vi "Scope_x410_2channel_IQ_PID.vi"() -> ()   [LabVIEW 2025]
uses:
  FPGA/DataMode.ctl
  <vilib>/Analysis/4window.llb/windowTd.ctl
  Host/Scope/controls/power_spectrum_unit.ctl
  Host/Scope5782/Scope/controls/5782_trigger_type.ctl
  Host/Scope/controls/Data_calc_mode.ctl
  Host/Scope/controls/Data_display_mode.ctl
  Host/Scope/controls/Graph_references.ctl
  Host/Scope/controls/graph_controls.ctl
  Host/Scope/controls/Channel_select_2fpga.ctl
  FPGA/PID/PID control enabled type.ctl
  <vilib>/userDefined/High Color/nirio_resource_hc.ctl
  Host/Scope/controls/All FP controls.ctl
  Host/Scope/controls/Output scale.ctl
  Host/Scope/controls/host_transfer_speed.ctl
  FPGA/cavity model/Piezo setting.ctl
  Host/Scope/controls/w12 scale.ctl
  Host/Scope/controls/FFT buffer type.ctl
  Host/Communication/Driver/RemoteConnection/RemoteReferences.ctl
  Host/FpgaRef/FpgaRef5761/ClockSource_5761.ctl
  Host/INI files/Settings file IQ PID/SettingsFileIQpid.lvclass
  C:/PXIe/InProgress/source/Host/INI files/Settings file base/SettingsFile.lvclass
  Host/Communication/Driver/RemoteConnection/RemoteConnection.lvclass
  Host/Scope/Scope5782_six_channel/Scope5782_six_channel.lvclass
  C:/PXIe/InProgress/source/Host/Scope/ScopeBase/ScopeBase.lvclass
  FPGA/fpga_settings.ctl
  Host/INI files/Settings file base/Save event.ctl
  Host/Scope/Scope5782_six_channel/Scope5782_six_channel.lvclass/Scope5782_six_channel.ctl
  Host/Scope/controls/ScopeMode.ctl
  Host/FpgaRef/FpgaRefx410/FpgaRefx410.lvclass
  C:/PXIe/InProgress/source/Host/FpgaRef/FpgaRefBase/FpgaRefBase.lvclass
  Host/FpgaRef/FpgaRef5761/FpgaRef5761.lvclass
  Host/Communication/global_stop.vi
  <vilib>/FPGAPlugInAG/USRP-X410/niLvFpga_Open_USRP-X410.vi
  <vilib>/rvi/interface/common/dynamic/niFpgaDynamicAddResources.vi
  <vilib>/Utility/error.llb/Error Cluster From Error Code.vi
  <vilib>/rvi/errors/niLvFpgaAdjustHostInterfaceError.vi
  Host/Communication/response.ctl
  Host/Communication/driver_status.ctl
  <vilib>/rvi/interface/nirviOpenFPGA/nirviOpenFPGA.xnode
  FPGA Bitfiles/FPGAmain_x410_IQ_PID_ek52GLrW3nU.lvbitx
  <vilib>/rvi/interface/nirviReadWriteControl/nirviReadWriteControl.xnode
  <vilib>/rvi/FXPMathLib/FxpInterpret/XNode/nifxpmath_Interpret.xnode
  C:/PXIe/InProgress/source/Host/FpgaRef/FpgaRefx410/FpgaRefx410.lvclass
  C:/PXIe/InProgress/source/Host/Scope/Scope5782_six_channel/Scope5782_six_channel.lvclass
  C:/PXIe/InProgress/source/Host/FpgaRef/FpgaRef5761/FpgaRef5761.lvclass
  Host/Communication/Driver/TcpServerDriver/TcpServerDriver.lvclass
  Host/Scope/ScopeBase/ScopeBase.lvclass
  Host/INI files/Settings file base/SettingsFile.lvclass
  <vilib>/FPGAPlugInAG/PXIe-7975R/niLvFpga_Open_PXIe-7975R.vi
  Host/FpgaRef/FpgaRefBase/FpgaRefBase.lvclass
  FPGA Bitfiles/FPGAmain_5761_zuew0qNtRjU.lvbitx
  NiFpgaLv.dll
  <vilib>/rvi/interface/Simulation/niFpgaSimulationCallBeginRW.vi
  <vilib>/Analysis/NI_AALPro.lvlib
panel:
  in  "Device Name":refnum<k15>="RIO0"
  in  "quench":bool
  out "Lower graph":dbl[][](graph)
  out "Upper graph":dbl[][](graph)
  out "Upper chart":dbl[][](graph)
  in  "Hold plot lower":bool caption="Hold plot"
  in  "Update once lower":bool
  in  "Hold plot upper":bool caption="Hold plot"
  in  "Update once upper":bool
  in  "FFT buffer size":T1
  in  "Transfer speed":T2
  out "All FP controls":T3
  in  "Show buffers":bool
  out "Adaptive FF graph":dbl[][](graph)
  in  "Tab Control":T4(tab)
  in  "b":fxp<+/-,16,2>
  in  "a":fxp<+/-,16,2>
  in  "Fequency [kHz]":dbl format="%#_8g"
  in  "I Feedback":T5
  in  "Ki*T AM":fxp<+/-,32,6> caption="Ki*T"
  in  "Kd/T AM":fxp<+/-,32,11> caption="Kd/T"
  in  "Kp AM":fxp<+/-,32,6> caption="Kp"
  in  "Feedback delay":u32
  in  "Trigger delay":u32
  in  "Acquire samples":u32
  in  "Kp Q":fxp<+/-,32,6> caption="Kp"
  in  "Kd/T  Q":fxp<+/-,32,11> caption="Kd/T"
  in  "Ki*T Q":fxp<+/-,32,6> caption="Ki*T"
  in  "Q Feedback":T5
  in  "Output gain dB":dbl
  in  "Host scale 5761":T6 caption="Host scale"
  in  "Input scale 5761":T6 caption="Input scale"
  in  "Host scale":T6
  in  "Input scale":T6
  in  "Output scale":T6
  in  "ch2 DC offset":dbl caption="DC offset\nChannel 2"
  in  "ch3 DC offset":dbl caption="DC offset\nChannel 3"
  in  "ch0 DC offset 2":dbl caption="DC offset\nChannel 0"
  in  "ch1 DC offset 2":dbl caption="DC offset\nChannel 1"
  in  "ch0 DC offset":dbl caption="DC offset\nChannel 0"
  in  "ch1 DC offset":dbl caption="DC offset\nChannel 1"
  in  "Setpoint":path
  in  "Feed forward":path
  in  "show setpoint":bool
  in  "show feedforward":bool
  in  "Setpoint enabled":bool
  in  "Piezo":T7
  in  "w0":dbl
  in  "Virtual cavity":bool
  in  "K2":dbl
  in  "Q2":dbl
  in  "w2":dbl
  in  "K3":dbl
  in  "Q3":dbl
  in  "w3":dbl
  in  "S":dbl=0.001 min=0.001 max=1000.0 format="%#_12g"
  in  "K1":dbl
  in  "Q1":dbl
  in  "w1":dbl
  in  "R1":dbl
  in  "w12":dbl format="%#_12g"
  in  "Cavity model":bool
  in  "Max output set":dbl min=0.0 max=16383.0
  out "Amp1":fxp<+,16,14>
  in  "Reset Quench Warning":bool
  in  "Measure Tau at Time":u32
  in  "Tau set":fxp<+/-,32,13>
  in  "Enable":bool
  out "Tau [µs]":fxp<+/-,64,26>
  out "Quench_Warning":bool
  out "Tau_set":fxp<+/-,32,13>
  in  "Input delay 5782":u32
  in  "Input delay 5761":u32
  in  "Count to skip 5782, stage 1":u32
  in  "Count to skip 5761, stage 1":u32
  in  "Count to skip 5782, stage 2":u32
  in  "Count to skip 5782, stage 3":u32
  in  "Count to skip 5761, stage 2":u32
  in  "Count to skip 5761, stage 3":u32
  in  "Vfi Vfq LP filter cut off frequency":dbl caption="MHz" min=0.0 max=10000.0
  in  "Vi Vq LP  filter cutoff fequency":dbl caption="MHz" min=0.0 max=10000.0
  in  "ch3 delay":dbl caption="ns" min=0.0 max=10000.0
  in  "ch1 delay":dbl caption="ns" min=0.0 max=10000.0
  in  "dw LP filter cut off frequency":dbl caption="MHz" min=0.0 max=10000.0
  in  "w12 LP  filter cutoff fequency":dbl caption="MHz" min=0.0 max=10000.0
  in  "dw scale":T8
  in  "w12 scale":T8
  in  "w12 - dt":dbl min=100.0 max=10000000.0
  in  "Calculate w12":bool
  in  "w12 - a":dbl format="%#_12g"
  in  "w12 - b":dbl
  in  "5761 resource":T9="PXI2Slot11"
  in  "Output enabled":bool=TRUE
  in  "Output delay delta":dbl(slide) scale=0.0..6.0
  in  "Output delay":dbl(slide) scale=0.0..6.0
  in  "Output mixer fequency [MHz]":dbl
  in  "Trigger":T10
  in  "Mode":T11
  in  "Mixer freq [MHz]":dbl
  in  "Unwrap phase":bool
  in  "#bins":i32=1 min=1 max=16
  in  "Unit":T12
  in  "Window":T13=1 items=["Rectangle"=0, "Hanning"=1, "Hamming"=2, "Blackman-Harris"=3, "Exact Blackman"=4, "Blackman"=5, "Flat Top"=6, "4 Term B-Harris "=7, "7 Term B-Harris"=8, "Low Sidelobe"=9, "Blackman Nuttall"=11, "Triangle"=30, "Bartlett-Hanning"=31, "Bohman"=32, "Parzen"=33, "Welch"=34, "Kaiser"=60, "Dolph-Chebyshev"=61, "Gaussian"=62]
  in  "Chart length":i32=400000
  in  "Trigmode":enum32{"Triggered", "Continuous"}(radio)
  in  "Reference for phase":T14
  in  "Graph_refs":T15
  out "Lower chart":dbl[][](graph)
  in  "Buffer":T17
  in  "Display":T18
  out "stop 2":bool
  in  "Zoom freq X":bool
  in  "Zoom freq Y":bool
  in  "Zoom time Y":bool
  in  "Zoom time X":bool
  in  "Samples per 5782 record":i32
  in  "Phase offset (deg)":dbl
  in  "Fequency [MHz]":dbl format="%#_8g"
  out "freqdata":cluster{"f0":dbl, "df":dbl, "magnitude":dbl[]}[](graph)
  in  "Rumode":bool
  in  "Singleshot":bool
  out "error IO":errorcluster
  in  "stop":bool
  # "FPGA setup"
  # "ns"
  # "Output delay"
  # "Auto Zoom"
  # "FFT"
  # "Auto Zoom"
  # "Delays"
  # "Amplitude modulation"
  # "x410"
  # "5761"
  # "5782"
  # "V"
  # "V"
  # "5761"
  # "V"
  # "V"
  # "V"
  # "V"
  # "Simulated data"
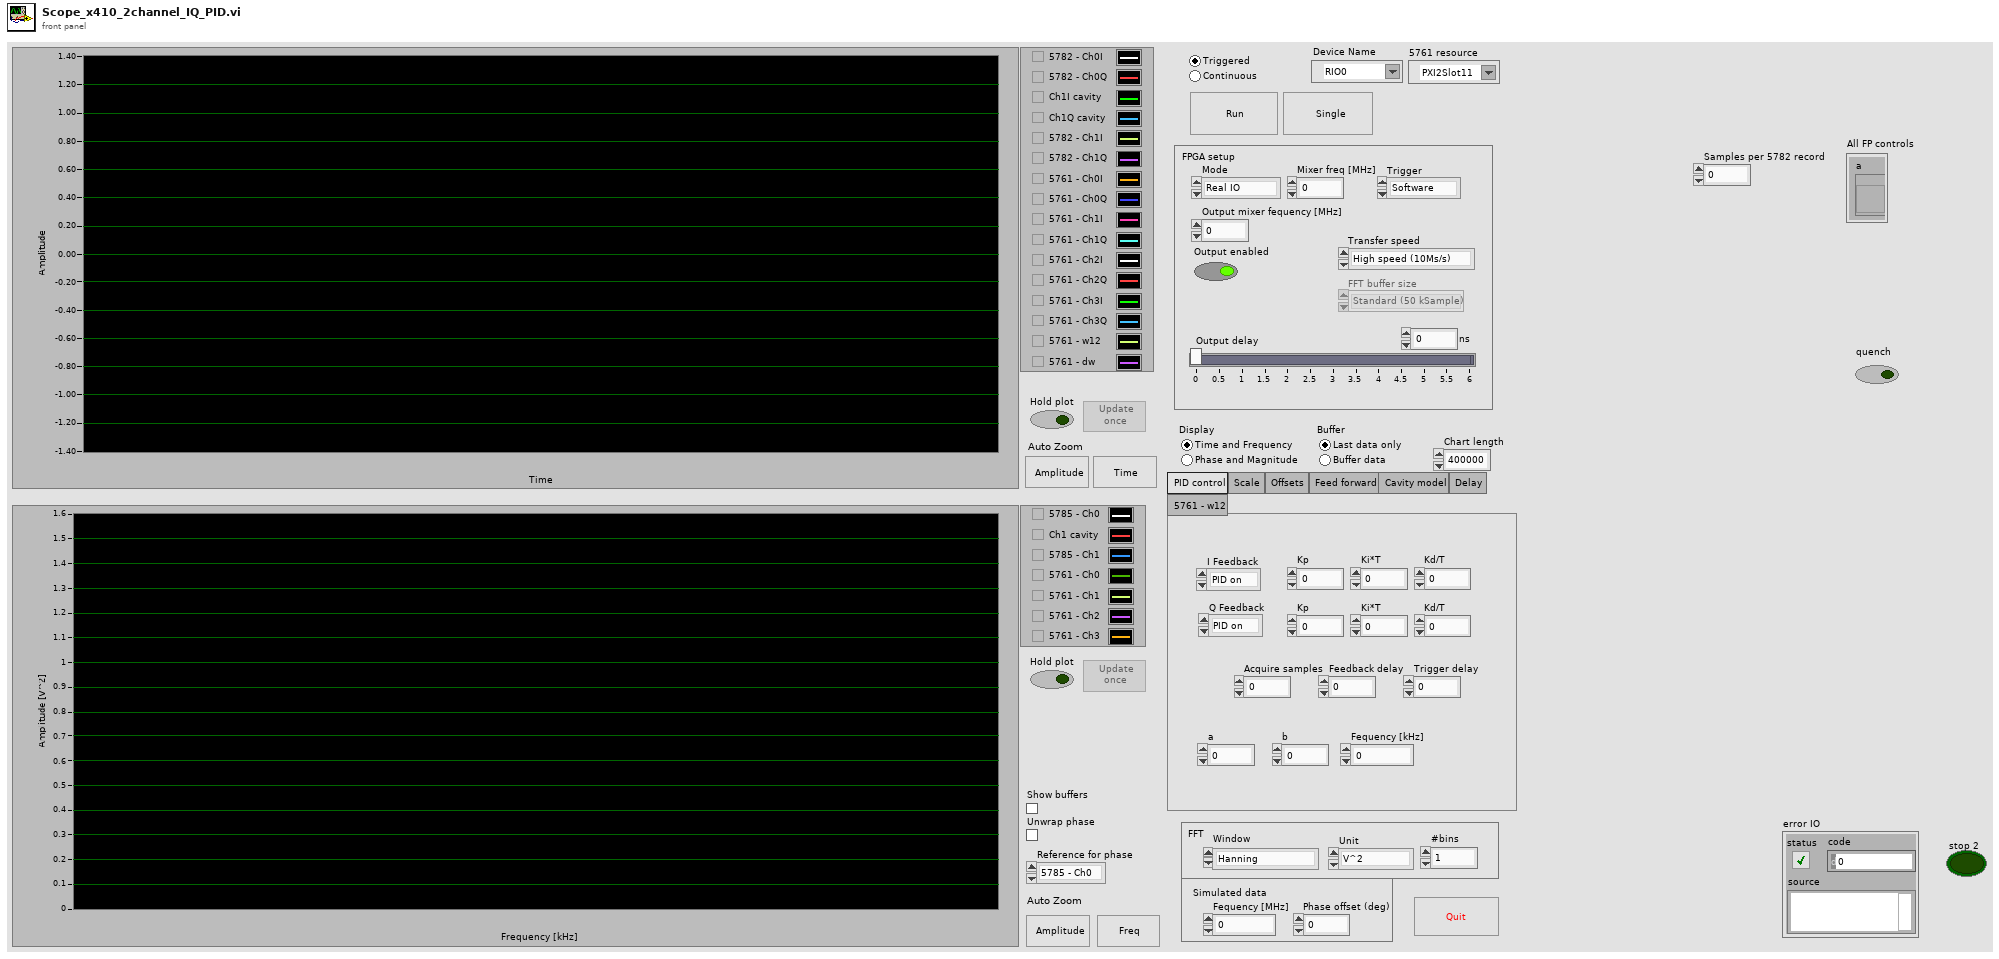
[diagram p1: front panel]
types:
  T1 = typedef "FFT buffer type.ctl" = enum16{"Standard (50 kSample)", "Long (250 kSample)"}
  T2 = typedef "host_transfer_speed.ctl" = enum16{"High speed (10Ms/s)", "Low speed (1Ms/s)", "Ultra low speed (50kS/s)"}
  T3 = typedef "All FP controls.ctl" = cluster{"ch1 DC offset":refnum<vi>, "ch0 DC offset":refnum<vi>, "ch1 DC offset 2":refnum<vi>, "ch0 DC offset 2":refnum<vi>, "ch3 DC offset":refnum<vi>, "ch2 DC offset":refnum<vi>, "Feedback Q":refnum<vi>, "Ki*T Q":refnum<vi>, "Kd/T  Q":refnum<vi>, "Kp Q":refnum<vi>, "Acquire samples":refnum<vi>, "Trigger delay":refnum<vi>, "Feedback delay":refnum<vi>, "Kp AM":refnum<vi>, "Kd/T AM":refnum<vi>, "Ki*T AM":refnum<vi>, "Feedback I":refnum<vi>, "#bins":refnum<vi>, "Window":refnum<vi>, "Unit":refnum<vi>, "Input delay 5761":refnum<vi>, "Input delay 5785":refnum<vi>, "S":refnum<vi>, "K1":refnum<vi>, "Q1":refnum<vi>, "R1":refnum<vi>, "w12":refnum<vi>, "Cavity model":refnum<vi>, "w1":refnum<vi>, "Mode":refnum<vi>, "Trigger":refnum<vi>, "Output mixer fequency [MHz]":refnum<vi>, "Output delay":refnum<vi>, "Mixer freq [MHz]":refnum<vi>, "Triggered":refnum<vi>, "Continuous":refnum<vi>, "Output scale":refnum<vi>, "Host scale":refnum<vi>, "Input scale":refnum<vi>, "IIR filter cutoff fequency [MHz]":refnum<vi>, "Host scale 5761":refnum<vi>, "Virtual cavity":refnum<vi>, "Input scale 5761":refnum<vi>, "Tranfer speed":refnum<vi>, "Count to skip 5782, stage 1":refnum<vi>, "Count to skip 5761, stage 1":refnum<vi>, "K2":refnum<vi>, "w2":refnum<vi>, "K3":refnum<vi>, "Q3":refnum<vi>, "Q2":refnum<vi>, "w3":refnum<vi>, "w0":refnum<vi>, "Piezo":refnum<vi>, "Measure Tau at Time":refnum<vi>, "Tau set":refnum<vi>, "Count to skip 5761, stage 2":refnum<vi>, "Count to skip 5761, stage 3":refnum<vi>, "Count to skip 5782, stage 2":refnum<vi>, "Count to skip 5782, stage 3":refnum<vi>, "Fequency [kHz]":refnum<vi>, "a":refnum<vi>, "b":refnum<vi>, "w12 - b":refnum<vi>, "w12 - a":refnum<vi>, "w12 - dt":refnum<vi>, "w12 scale":refnum<vi>, "dw scale":refnum<vi>, "w12 LP  filter cutoff fequency":refnum<vi>, "dw LP filter cut off frequency":refnum<vi>, "ch1 delay":refnum<vi>, "ch3 delay":refnum<vi>, "Vi Vq LP  filter cutoff fequency":refnum<vi>, "Vfi Vfq LP filter cut off frequency":refnum<vi>}
  T4 = enum32{"PID control", "Scale", "Offsets", "Feed forward", "Cavity model", "Quench", "Delay", "5761 - w12"}
  T5 = typedef "PID control enabled type.ctl" = enum16{"PID on", "Ref", "Zero"}
  T6 = typedef "Output scale.ctl" = enum16{"x1", "x2", "x4", "x8", "x16", "x32"}
  T7 = typedef "Piezo setting.ctl" = enum16{"Off", "On - Ch 0", "On - Ch 1"}
  T8 = typedef "w12 scale.ctl" = enum16{"x1", "1/2", "1/4", "1/8", "1/16", "1/32", "1/64", "1/128", "1/256", "1/512", "1/1024", "1/2048", "1/4096", "1/8192"}
  T9 = typedef "nirio_resource_hc.ctl" = tag
  T10 = typedef "5782_trigger_type.ctl" = enum16{"Software", "Trigger input"}
  T11 = typedef "DataMode.ctl" = enum16{"Real IO", "Simulated"}
  T12 = typedef "power_spectrum_unit.ctl" = enum16{"V^2", "V", "dBV"}
  T13 = typedef "NI_AALPro.lvlib/windowTd.ctl" = u32
  T14 = typedef "Channel_select_2fpga.ctl" = enum16{"5785 - Ch0", "5785 - Ch1 cavity", "5785 - Ch1", "5761 - Ch0", "5761 - Ch1", "5761 - Ch2", "5761 - Ch3"}
  T15 = typedef "Graph_references.ctl" = cluster{"upper":T16, "lower":T16, "Freq graph":refnum<vi>, "Adaptive FF graph":refnum<vi>}
  T16 = typedef "graph_controls.ctl" = cluster{"Graph":refnum<vi>, "Time btn":refnum<vi>, "Amplitude btn":refnum<vi>, "Chart":refnum<vi>}
  T17 = typedef "Data_display_mode.ctl" = enum32{"Last data only", "Buffer data"}
  T18 = typedef "Data_calc_mode.ctl" = enum32{"Time and Frequency", "Phase and Magnitude"}
  T19 = typedef "ClockSource_5761.ctl" = enum8{"Internal Clock PLL Off", "Internal Clock PLL On (CLK_IN)", "External Clock (CLK_IN)", "Internal Clock PLL On (IoModSyncClk)", "External Clock (IoModSyncClk)"}
  T20 = typedef "RemoteConnection.lvclass/RemoteReferences.ctl" = cluster{"a":refnum<vi>, "b":refnum<vi>, "fm":refnum<vi>, "Output delay":refnum<vi>, "Output delay delta":refnum<vi>}
  T21 = typedef "response.ctl" = cluster{"driver status":T22, "Sender":string, "Type":i32, "Variant":variant}
  T22 = typedef "driver_status.ctl" = enum16{"Normal", "Startup", "Connection lost", "Reconnected", "Timeout", "Idle", "Busy"}
  T23 = typedef "message_queue.ctl" = refnum<queue>
  T24 = typedef "INI Save Event.ctl" = refnum<user-event>
  T25 = typedef "Save event.ctl" = cluster{"Automatic":bool, "Save":bool}
  T26 = typedef "fpga_settings.ctl" = enum16{"Feedback Enable", "New FIR coeffs", "FIR shift", "Enable filter", "Set Downsample", "Downsample", "CIC Gain", "Record length", "Trigger samples", "Quiet time", "a_am", "b_am", "Use fixed delay", "fixed sin_fi", "fixed cos_fi", "Ki*Tau", "Kp", "Kd_Tau", "Fi_start", "Fi_delta", "DC_offs 0", "DC_offs 1", "DC_offs 2", "DC_offs 3", "Ki*Tau am", "Kp am", "Kd_Tau am", "Feedback AM", "Trigger delay", "Feedback delay", "Setpoint enable", "Beam enable", "Samples to acquire", "Cavity Enable", "Cavity C1", "Cavity C2", "Cavity C3", "Cavity C4", "Cavity C5", "Input delay", "Ki*Tau Q", "Kp Q", "Kd_Tau Q", "Adaptive FF enable", "Feedforward a0", "Feedforward b0", "FF src adress", "FF dest adress", "Output scale", "Input scale", "Host scale", "FF_IIR b0", "FF_IIR b1", "FF_IIR b2", "FF_IIR-a1", "FF_IIR-a2", "Enable HW trigger", "Virtual cavity", "Samples to skip", "Samples to skip 2", "Samples to skip 3", "Cavity C3_2", "Cavity C4_2", "Cavity C5_2", "Cavity C3_3", "Cavity C4_3", "Cavity C5_3", "Cavity_w0_dt", "Piezo setting", "Quench t0", "Quench tau set", "Quench enabled", "Quench reset", "PID enabled I", "PID enabled Q", "Cavity filter a", "Cavity filter b", "Disable e(n)", "FF e(n) src address", "FF first address", "FF last address", "FF PID first address", "FF PID last address", "Amp IIR b0", "Amp IIR b1", "Amp IIR b2", "Amp IIR-a1", "Amp IIR-a2", "Adaptation factor", "Inv Amp LP b0", "Inv Amp LP b1", "Inv Amp LP b2", "Inv Amp LP-a1", "Inv Amp LP-a2", "Inv Amp c0", "Inv Amp c1", "Inv Amp c2", "Inv Amp c3", "Inv Amp c4", "Inv Amp -d1", "Inv Amp -d2", "Inv Amp -d3", "Inv Amp -d4", "w12_a", "w12_b", "w12_dt", "w12_scale", "dw_scale", "Extra output select", "Extra fi sin", "Extra fi cos", "Extra output scale", "Quench max output"}
  T27 = enum8{"Enabled", "Disabled", "Disabled and Grayed Out"}
  T28 = typedef "ScopeMode.ctl" = enum16{"Stopped", "Single", "Running", "Continuous"}
  T29 = typedef "PlotUpdate type.ctl" = enum16{"None", "Graph", "Chart", "Freq"}
  T30 = typedef "Feedforward.ctl" = cluster{"Beam I":dbl[], "Beam Q":dbl[], "Feedforward I":dbl[], "Feedforward Q":dbl[], "Setpoint I":dbl[], "Setpoint Q":dbl[]}
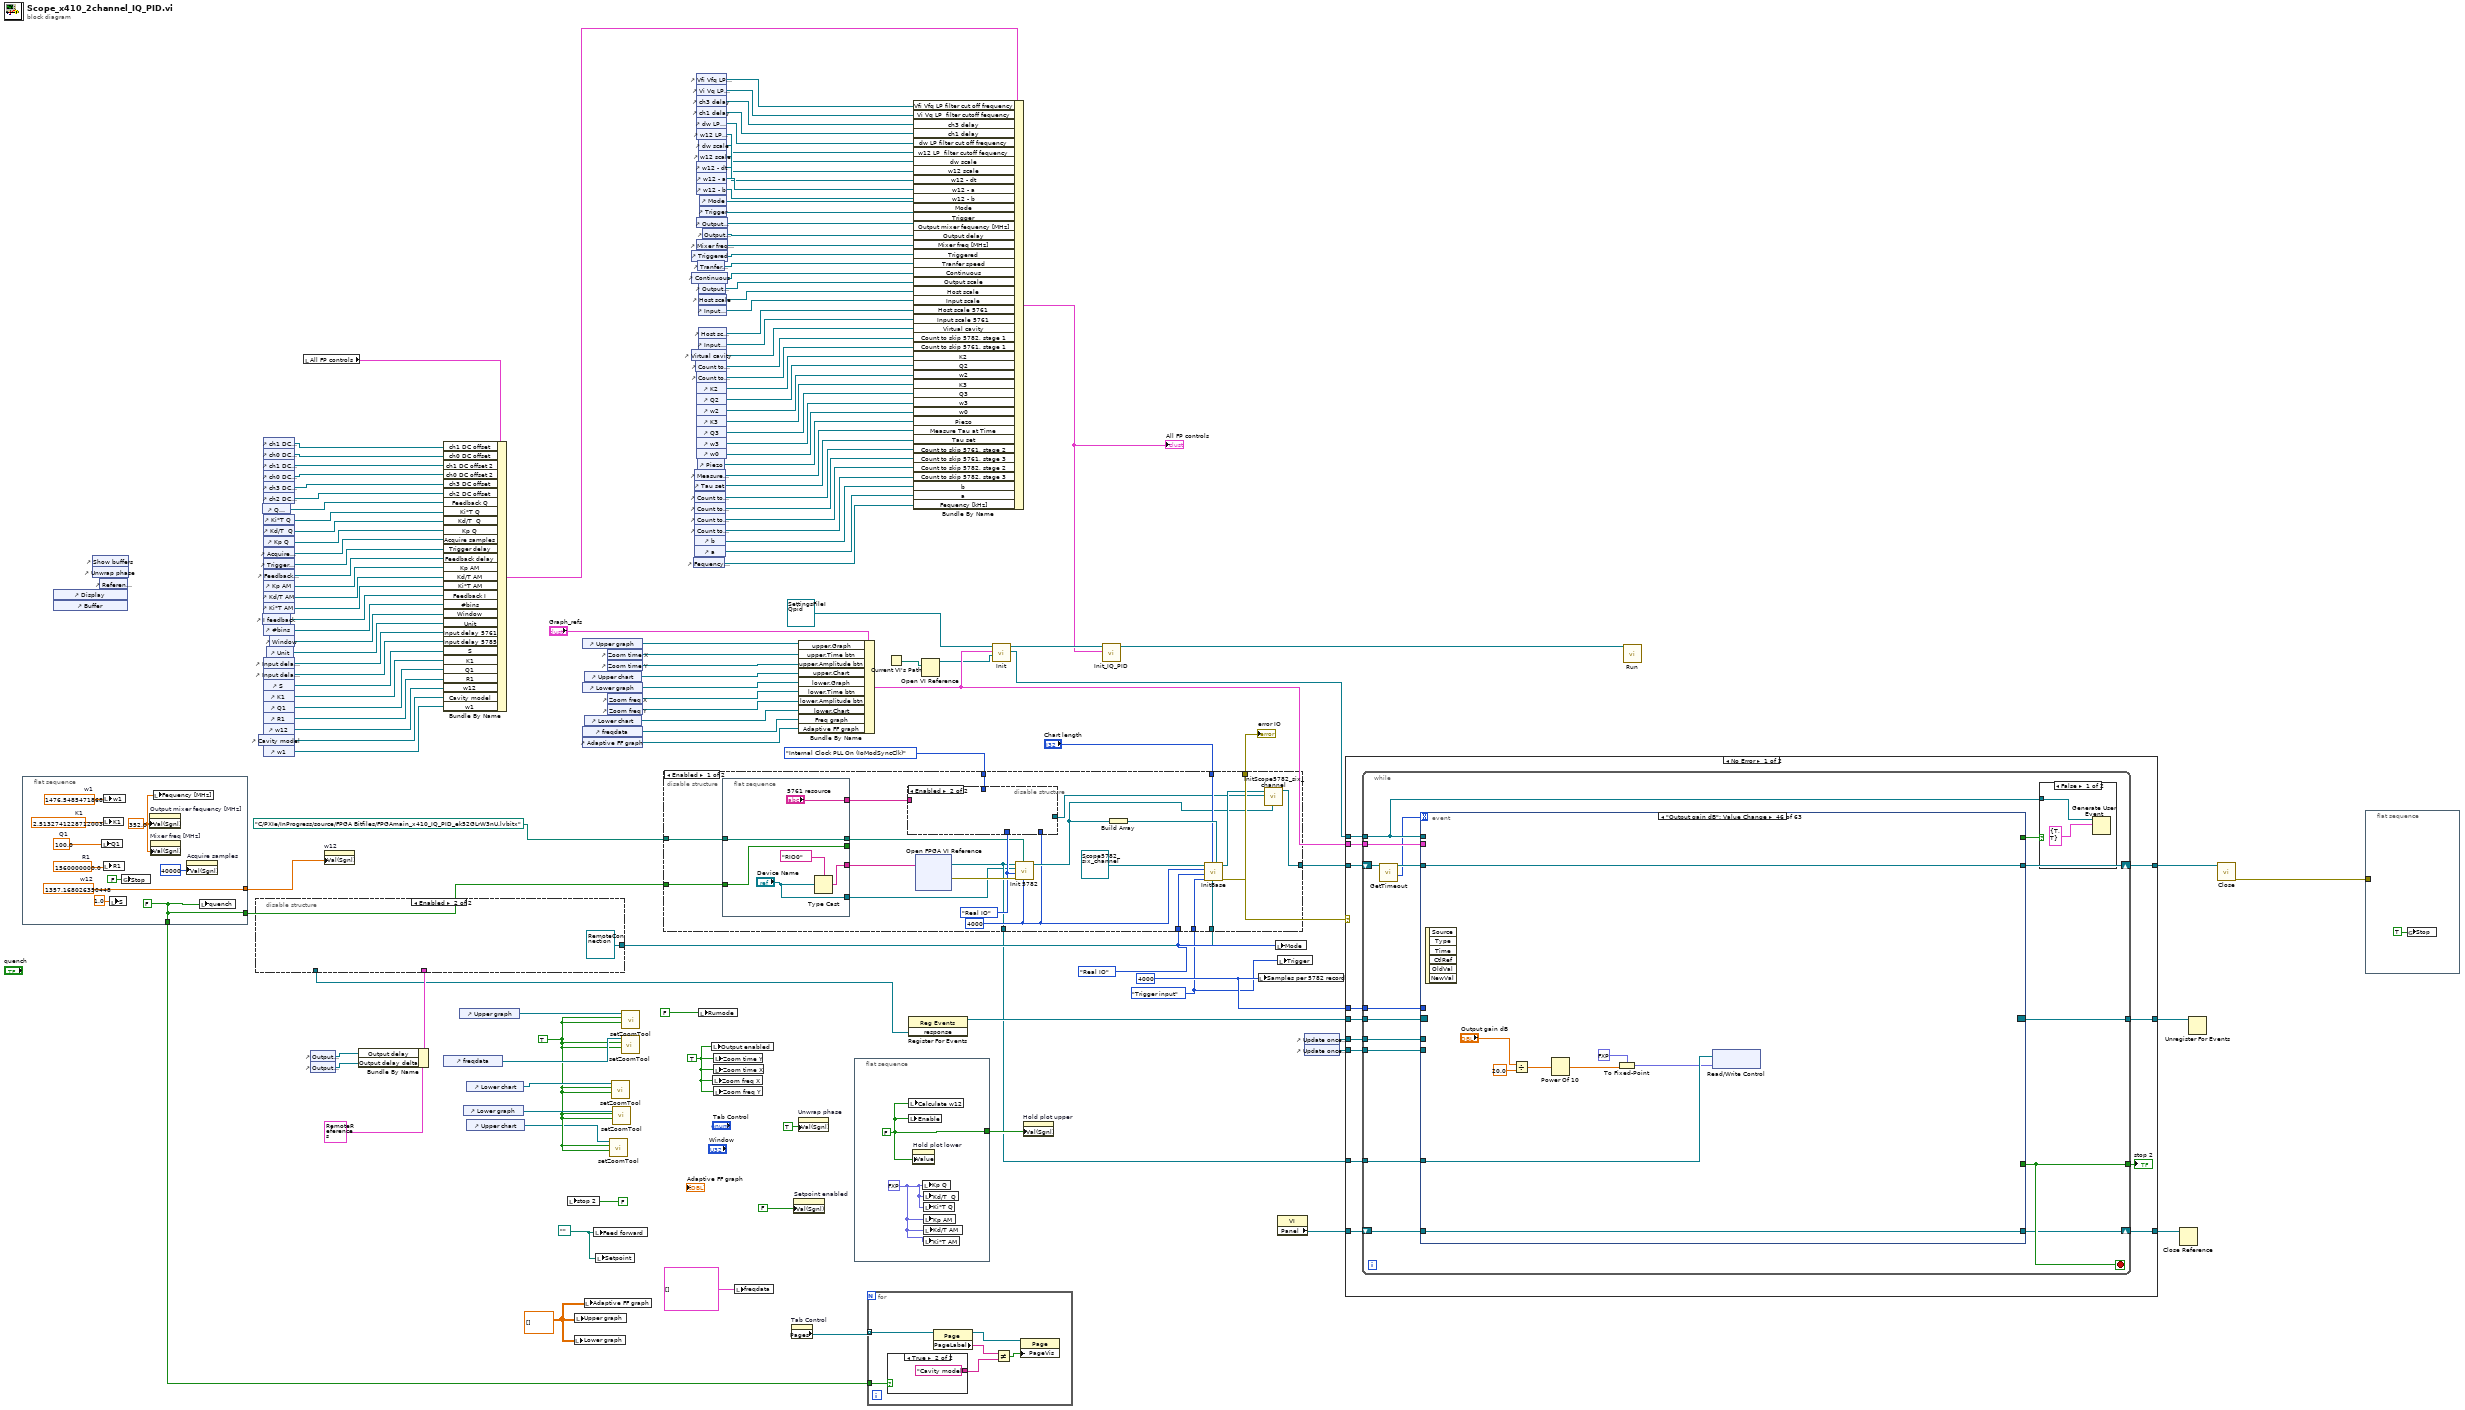
[diagram p0: block diagram]
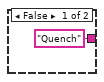
[diagram p2: hidden frame]
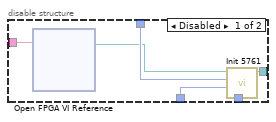
[diagram p3: hidden frame]
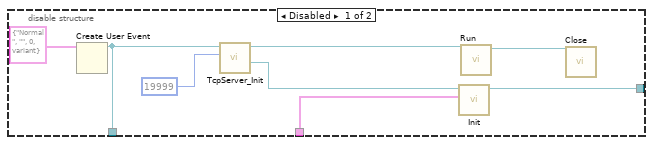
[diagram p5: hidden frame]
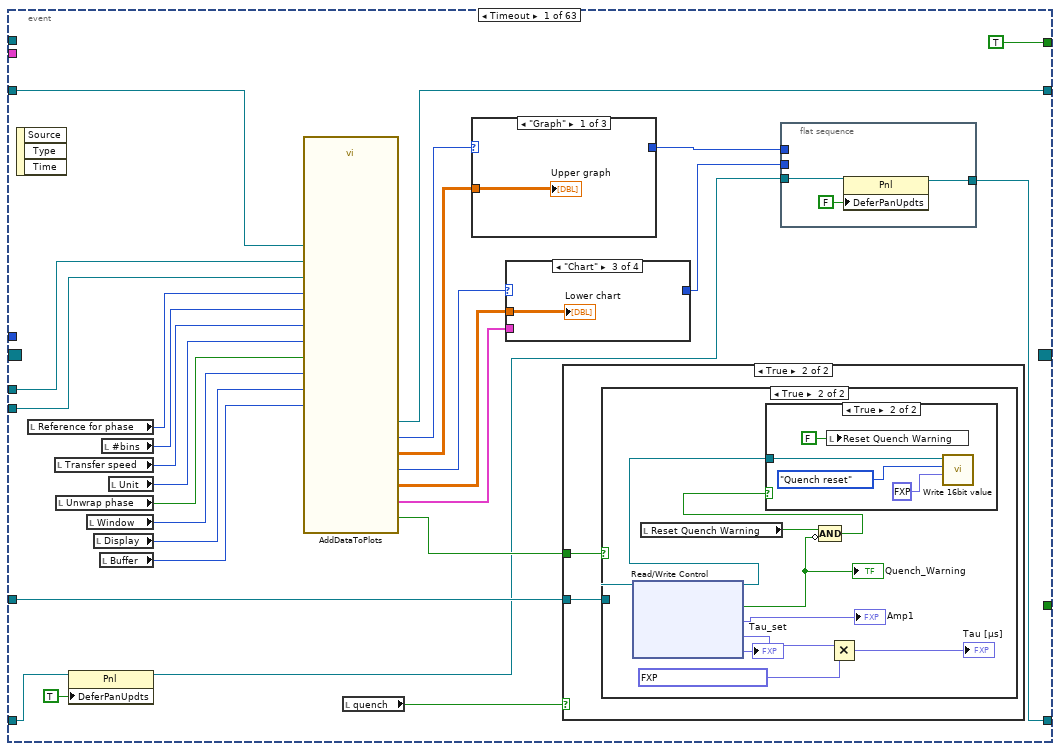
[diagram p7: hidden frame]
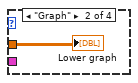
[diagram p12: hidden frame]
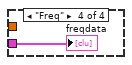
[diagram p13: hidden frame]
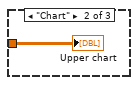
[diagram p14: hidden frame]
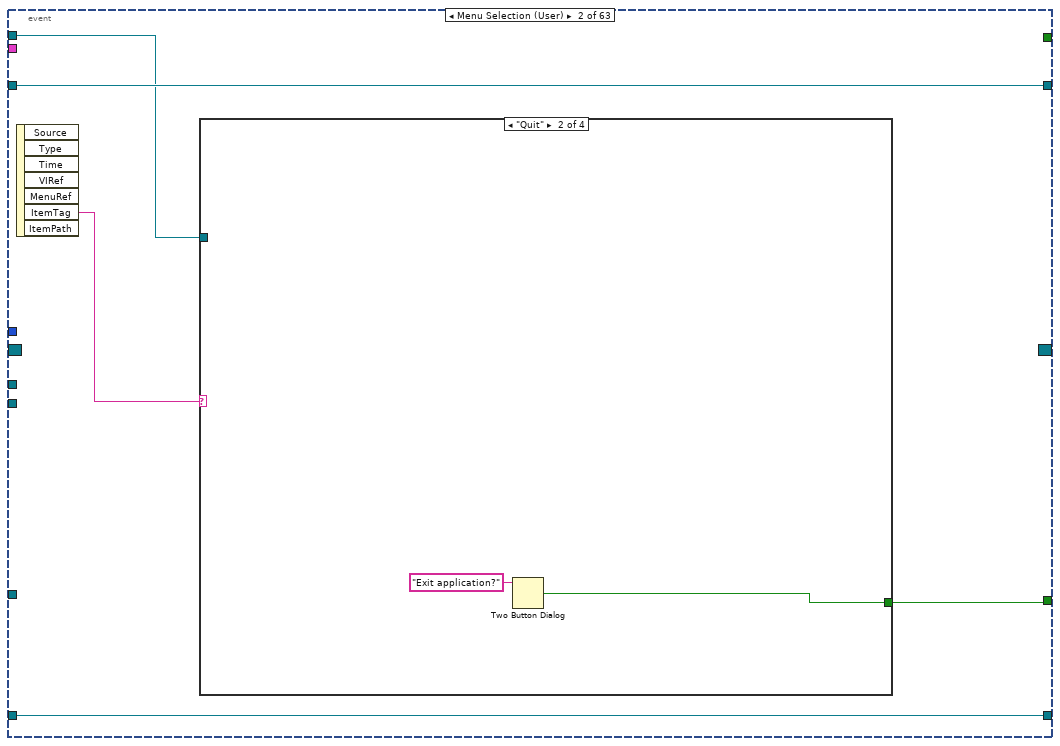
[diagram p16: hidden frame]
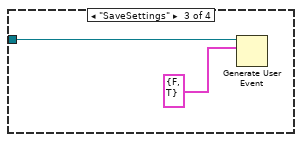
[diagram p18: hidden frame]
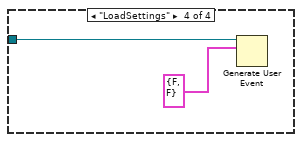
[diagram p19: hidden frame]
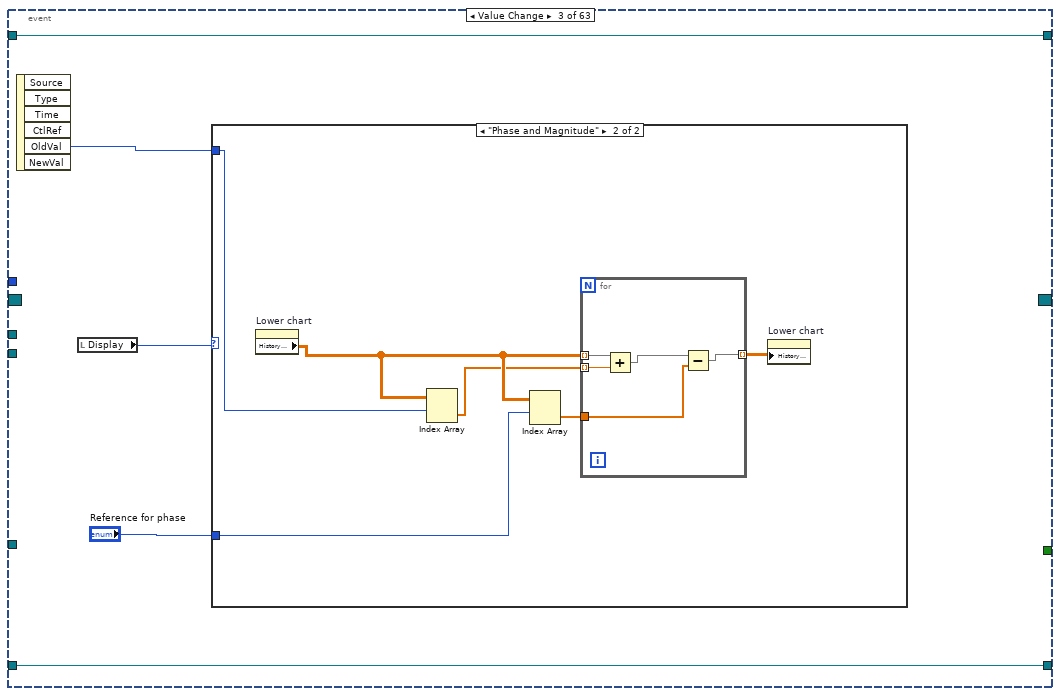
[diagram p20: hidden frame]
diagram:
  w107 = DataMode."Real IO" ("Mode")
  w109 = path "" ("Feed forward")
  w106 = 5782_trigger_type."Trigger input" ("Trigger")
  w21 = TRUE ("Zoom  X")
  w113 = TRUE ("Rumode")
  w112 = 4000 ("Samples to aqcuire")
  w23 = dbl[][] [] ("Timedata")
  n1 = flat-sequence {
    tunnel: [w141] -> w54
    tunnel: [w138] -> w16
    tunnel: [w138] -> w15
    frame #0 {
      w138 = FALSE ("quench")
      w139 = 352.0 ("Value (Signaling)")
      w143 = 2.5132741228712003  # K1
      w142 = 100.0  # Q1
      w144 = 1476.54854718683  # w1
      w145 = 1560000000.0  # R1
      w141 = 1357.168026350448  # w12
      n2 = local write "Q1"(w142) -> ()
      n3 = local write "w1"(w144) -> ()
      n4 = local write "K1"(w143) -> ()
      n5 = local write "R1"(w145) -> ()
      n6 = local write "S"(1.0 ("S")) -> ()
      n7 = global write "global_stop.vi" "Stop"(FALSE ("Stop")) -> ()
      n8 = property on="Output mixer fequency [MHz]" class="DigNum (strict)"("Val(Sgnl)"=w139) -> ()  [unwired: 2 in, 2 out]
      n9 = property on="Mixer freq [MHz]" class="DigNum (strict)"("Val(Sgnl)"=w139) -> ()  [unwired: 2 in, 2 out]
      n10 = local write "Fequency [MHz]"(w139) -> ()
      n11 = property on="Acquire samples" class="DigNum (strict)"("Val(Sgnl)"=u32 40000 ("Value (Signaling)")) -> ()  [unwired: 2 in, 2 out]
      n12 = local write "quench"(w138) -> ()
    }
  }
  n13 = control-ref of="Display"() -> ()  [unwired: 1 out]
  n14 = control-ref of="Buffer"() -> ()  [unwired: 1 out]
  n15 = control-ref of="Show buffers"() -> ()  [unwired: 1 out]
  n16 = control-ref of="Unwrap phase"() -> ()  [unwired: 1 out]
  n17 = control-ref of="Reference for phase"() -> ()  [unwired: 1 out]
  n18 = control-ref of="Cavity model"() -> (w71:refnum<vi>)
  n19 = control-ref of="Q Feedback"() -> (w92:refnum<vi>)
  n20 = control-ref of="I feedback"() -> (w82:refnum<vi>)
  n21 = control-ref of="Ki*T Q"() -> (w91:refnum<vi>)
  n22 = control-ref of="Kd/T  Q"() -> (w90:refnum<vi>)
  n23 = control-ref of="Kp Q"() -> (w89:refnum<vi>)
  n24 = control-ref of="Acquire samples"() -> (w88:refnum<vi>)
  n25 = control-ref of="Trigger delay"() -> (w87:refnum<vi>)
  n26 = control-ref of="Feedback delay"() -> (w86:refnum<vi>)
  n27 = control-ref of="Kp AM"() -> (w85:refnum<vi>)
  n28 = control-ref of="Kd/T AM"() -> (w84:refnum<vi>)
  n29 = control-ref of="Ki*T AM"() -> (w83:refnum<vi>)
  n30 = control-ref of="#bins"() -> (w81:refnum<vi>)
  n31 = control-ref of="Input delay 5761"() -> (w78:refnum<vi>)
  n32 = control-ref of="Input delay 5782"() -> (w77:refnum<vi>)
  n33 = control-ref of="S"() -> (w76:refnum<vi>)
  n34 = control-ref of="K1"() -> (w75:refnum<vi>)
  n35 = control-ref of="Q1"() -> (w74:refnum<vi>)
  n36 = control-ref of="R1"() -> (w73:refnum<vi>)
  n37 = control-ref of="w12"() -> (w72:refnum<vi>)
  n38 = control-ref of="w1"() -> (w70:refnum<vi>)
  n39 = control-ref of="ch1 DC offset"() -> (w98:refnum<vi>)
  n40 = control-ref of="ch0 DC offset"() -> (w97:refnum<vi>)
  n41 = control-ref of="ch1 DC offset 2"() -> (w96:refnum<vi>)
  n42 = control-ref of="ch0 DC offset 2"() -> (w95:refnum<vi>)
  n43 = control-ref of="ch3 DC offset"() -> (w94:refnum<vi>)
  n44 = control-ref of="ch2 DC offset"() -> (w93:refnum<vi>)
  n45 = control-ref of="Unit"() -> (w79:refnum<vi>)
  n46 = control-ref of="Window"() -> (w80:refnum<vi>)
  n47 = local read "All FP controls"() -> (w99:T3)
  n48 = control-ref of="Output delay"() -> (w116:refnum<vi>)
  n49 = control-ref of="Output delay delta"() -> (w115:refnum<vi>)
  n50 = property on="w12" class="DigNum (strict)"("Val(Sgnl)"=w54) -> ()  [unwired: 2 in, 2 out]
  n51 = Bundle By Name(cluster=T20 {"a"=refnum, "b"=refnum, "fm"=refnum, "Output delay"=refnum, "Output delay delta"=refnum} ("refs"), "Output delay"=w116, "Output delay delta"=w115) -> (w120:T20)
  n52 = disable-structure shown="Enabled" {
    disable-tunnel: w120 -> [w154 _]
    disable-tunnel: [w149 _] -> w118
    disable-tunnel: [w147 refnum<class "RemoteConnection.lvclass"> refnum ("RemoteConnection")] -> w105
    frame Disabled {
      n53 = Create User Event(user event datatype=T21 {"driver status"=enum."Normal", "Sender"="", "Type"=0, "Variant"=variant} ("response")) -> (user event=w149:refnum<user-event>)  [unwired: 1 in, 1 out]
      n54 = call "TcpServer_Init.vi"("local port"=u16 19999, "response event"=w149) -> ("Message queue"=w153:T23, "TcpServerDriver"=w151:refnum<class "TcpServerDriver.lvclass">)  [unwired: 8 in]
      n55 = call "Init.vi"("refs"=w154, "server queue"=w153) -> ("RemoteConnection"=w147:refnum<class "RemoteConnection.lvclass">)  [unwired: 9 in]
      n56 = call-dynamic "Run.vi"("BaseDriver in"=w151) -> ("BaseDriver out"=w152:refnum<class "TcpServerDriver.lvclass">)  [unwired: 9 in, 1 out]
      n57 = call-dynamic "Close.vi"("BaseDriver in"=w152) -> ()  [unwired: 9 in, 2 out]
    }
    frame Enabled {
    }
  }
  n58 = control-ref of="freqdata"() -> (w131:refnum<vi>)
  n59 = Bundle By Name(cluster=w99, "ch1 DC offset"=w98, "ch0 DC offset"=w97, "ch1 DC offset 2"=w96, "ch0 DC offset 2"=w95, "ch3 DC offset"=w94, "ch2 DC offset"=w93, "Feedback Q"=w92, "Ki*T Q"=w91, "Kd/T  Q"=w90, "Kp Q"=w89, "Acquire samples"=w88, "Trigger delay"=w87, "Feedback delay"=w86, "Kp AM"=w85, "Kd/T AM"=w84, "Ki*T AM"=w83, "Feedback I"=w82, "#bins"=w81, "Window"=w80, "Unit"=w79, "Input delay 5761"=w78, "Input delay 5785"=w77, "S"=w76, "K1"=w75, "Q1"=w74, "R1"=w73, "w12"=w72, "Cavity model"=w71, "w1"=w70) -> (w69:T3)
  n60 = control-ref of="Upper graph"() -> (w132:refnum<vi>)
  n61 = control-ref of="Lower graph"() -> (w22:refnum<vi>)
  n62 = control-ref of="Lower chart"() -> (w117:refnum<vi>)
  n63 = control-ref of="Upper chart"() -> (w20:refnum<vi>)
  n64 = local write "stop 2"(FALSE ("stop 2")) -> ()
  n65 = local write "Lower graph"(w23) -> ()
  n66 = local write "Upper graph"(w23) -> ()
  n67 = control-ref of="Upper graph"() -> (w129:refnum<vi>)
  n68 = control-ref of="Lower graph"() -> (w125:refnum<vi>)
  n69 = control-ref of="freqdata"() -> (w121:refnum<vi>)
  n70 = control-ref of="Adaptive FF graph"() -> (w100:refnum<vi>)
  n71 = control-ref of="Upper chart"() -> (w126:refnum<vi>)
  n72 = control-ref of="Lower chart"() -> (w122:refnum<vi>)
  n73 = local write "Adaptive FF graph"(w23) -> ()
  n74 = local write "Feed forward"(w109) -> ()
  n75 = local write "Setpoint"(w109) -> ()
  n76 = control-ref of="Zoom time X"() -> (w128:refnum<vi>)
  n77 = control-ref of="Zoom time Y"() -> (w127:refnum<vi>)
  n78 = control-ref of="Zoom freq X"() -> (w124:refnum<vi>)
  n79 = control-ref of="Zoom freq Y"() -> (w123:refnum<vi>)
  n80 = call "setZoomTool.vi"("Zoom Y"=w21, "Zoom  X"=w21, "reference"=w20) -> ()  [unwired: 9 in]
  n81 = call "setZoomTool.vi"("Zoom Y"=w21, "Zoom  X"=w21, "reference"=w117) -> ()  [unwired: 9 in]
  n82 = call "setZoomTool.vi"("Zoom Y"=w21, "Zoom  X"=w21, "reference"=w22) -> ()  [unwired: 9 in]
  n83 = call "setZoomTool.vi"("Zoom Y"=w21, "Zoom  X"=w21, "reference"=w131) -> ()  [unwired: 9 in]
  n84 = call "setZoomTool.vi"("Zoom Y"=w21, "Zoom  X"=w21, "reference"=w132) -> ()  [unwired: 9 in]
  n85 = disable-structure shown="Enabled" {
    disable-tunnel: ClockSource_5761."Internal Clock PLL On (IoModSyncClk)" ("Clock Source") -> [w177 _]
    disable-tunnel: w107 -> [w173 _]
    disable-tunnel: w106 -> [w172 _]
    disable-tunnel: w105 -> [w171 _]
    disable-tunnel: "Chart length" -> [w170 _]
    disable-tunnel: [w169 _] -> w52
    disable-tunnel: [w165 _] -> w101
    disable-tunnel: [w159 _] -> w1
    disable-tunnel: w15 -> [w160 _]
    disable-tunnel: path "C:/PXIe/InProgress/source/FPGA Bitfiles/FPGAmain_x410_IQ_PID_ek52GLrW3nU.lvbitx" -> [w157 _]
    frame Enabled {
      w161 = u16 4000 ("Samples to aqcuire")
      w162 = DataMode."Real IO" ("Mode")
      n86 = flat-sequence {
        tunnel: ["5761 resource"] -> w175
        tunnel: [w186] -> w174
        tunnel: [w188] -> _
        tunnel: w160 -> [w188]
        tunnel: [w185] -> w158
        tunnel: w157 -> [w185]
        tunnel: ["Device Name"] -> w156
        frame #0 {
          n87 = Type Cast(type=tag "RIO0" ("resource name"), x="Device Name") -> (*(type *) &x=w186:tag)
        }
      }
      n88 = disable-structure shown="Enabled" {
        disable-tunnel: w177 -> [w183 _]
        disable-tunnel: w175 -> [w182 _]
        disable-tunnel: [w181 _] -> w163
        disable-tunnel: w162 -> [w180 _]
        disable-tunnel: w161 -> [w179 _]
        frame Disabled {
          n89 = xnode "Open FPGA VI Reference"("resource name"=w182) -> ("FPGA VI Reference Out"=w178:refnum<k20>)  [unwired: 1 in, 1 out]
          n90 = call "Init 5761.vi"("Record length"=w179, "Mode"=w180, "Clock Source"=w183, "FPGA ref"=w178) -> ("FpgaRef5761 out"=w181:refnum<class "FpgaRef5761.lvclass">)  [unwired: 6 in, 1 out]
        }
        frame Enabled {
        }
      }
      n91 = xnode "Open FPGA VI Reference"("resource name"=w174) -> ("FPGA VI Reference Out"=w159:refnum<k20>, "error out"=w167:errorcluster)  [unwired: 1 in]
      n92 = call "Init 5782.vi"("Record length"=w161, "bitfile path"=w158, "error in (no error)"=w167, "Mode"=w162, "Device Name"=w156, "FPGA ref"=w159) -> ("FpgaRef5782 Out"=w164:refnum<class "FpgaRefx410.lvclass">)  [unwired: 4 in, 1 out]
      n93 = Build Array(w164) -> (w176:refnum<class "FpgaRefx410.lvclass">[])
      n94 = call "InitBase.vi"("FPGA refs"=w176, "RemoteConnection"=w171, "Chart length"=w170, "Trigger"=w172, "data mode"=w173, "Samples Per Trigger"=w161, "ScopeBase in"=refnum<class "Scope5782_six_channel.lvclass"> refnum ("Scope5761")) -> ("error out"=w169:errorcluster, "ScopeBase out"=w166:refnum<class "Scope5782_six_channel.lvclass">)  [unwired: 3 in]
      n95 = call "InitScope5782_six_channel.vi"("FpgaRef5782"=w164, "FpgaRef5761"=w163, "Scope5785_six_channel"=w166) -> ("Scope5785_six_channel out"=w165:refnum<class "Scope5782_six_channel.lvclass">)  [unwired: 7 in, 1 out]
    }
    frame Disabled {
    }
  }
  "error IO" <- w52
  n96 = control-ref of="Virtual cavity"() -> (w47:refnum<vi>)
  n97 = control-ref of="Triggered"() -> (w63:refnum<vi>)
  n98 = control-ref of="Continuous"() -> (w62:refnum<vi>)
  n99 = control-ref of="Fequency [kHz]"() -> (w17:refnum<vi>)
  n100 = control-ref of="a"() -> (w18:refnum<vi>)
  n101 = control-ref of="Measure Tau at Time"() -> (w31:refnum<vi>)
  n102 = control-ref of="Tau set"() -> (w30:refnum<vi>)
  n103 = control-ref of="Count to skip 5761, stage 2"() -> (w29:refnum<vi>)
  n104 = control-ref of="Count to skip 5761, stage 3"() -> (w28:refnum<vi>)
  n105 = control-ref of="Count to skip 5782, stage 2"() -> (w27:refnum<vi>)
  n106 = control-ref of="Count to skip 5782, stage 3"() -> (w26:refnum<vi>)
  n107 = control-ref of="b"() -> (w19:refnum<vi>)
  n108 = control-ref of="Count to skip 5782, stage 1"() -> (w43:refnum<vi>)
  n109 = control-ref of="Vfi Vfq LP filter cut off frequency"() -> (w3:refnum<vi>)
  n110 = control-ref of="Vi Vq LP  filter cutoff fequency"() -> (w4:refnum<vi>)
  n111 = control-ref of="ch3 delay"() -> (w5:refnum<vi>)
  n112 = control-ref of="ch1 delay"() -> (w6:refnum<vi>)
  n113 = control-ref of="dw LP filter cut off frequency"() -> (w7:refnum<vi>)
  n114 = control-ref of="w12 LP  filter cutoff fequency"() -> (w8:refnum<vi>)
  n115 = control-ref of="w12 - dt"() -> (w11:refnum<vi>)
  n116 = control-ref of="w12 - a"() -> (w12:refnum<vi>)
  n117 = control-ref of="w12 - b"() -> (w13:refnum<vi>)
  n118 = control-ref of="Count to skip 5761, stage 1"() -> (w42:refnum<vi>)
  n119 = control-ref of="K2"() -> (w41:refnum<vi>)
  n120 = control-ref of="Q2"() -> (w40:refnum<vi>)
  n121 = control-ref of="w2"() -> (w39:refnum<vi>)
  n122 = control-ref of="K3"() -> (w38:refnum<vi>)
  n123 = control-ref of="Q3"() -> (w37:refnum<vi>)
  n124 = control-ref of="w3"() -> (w36:refnum<vi>)
  n125 = control-ref of="w0"() -> (w35:refnum<vi>)
  n126 = control-ref of="Output mixer fequency [MHz]"() -> (w66:refnum<vi>)
  n127 = control-ref of="Mixer freq [MHz]"() -> (w64:refnum<vi>)
  n128 = control-ref of="Tranfer speed"() -> (w46:refnum<vi>)
  n129 = control-ref of="Piezo"() -> (w34:refnum<vi>)
  n130 = control-ref of="Output scale"() -> (w53:refnum<vi>)
  n131 = control-ref of="dw scale"() -> (w9:refnum<vi>)
  n132 = control-ref of="w12 scale"() -> (w10:refnum<vi>)
  n133 = control-ref of="Host scale"() -> (w51:refnum<vi>)
  n134 = control-ref of="Input scale"() -> (w50:refnum<vi>)
  n135 = control-ref of="Host scale 5761"() -> (w49:refnum<vi>)
  n136 = control-ref of="Input scale 5761"() -> (w48:refnum<vi>)
  n137 = local write "Rumode"(FALSE ("Rumode")) -> ()
  n138 = control-ref of="Mode"() -> (w68:refnum<vi>)
  n139 = control-ref of="Trigger"() -> (w67:refnum<vi>)
  n140 = control-ref of="Output delay"() -> (w65:refnum<vi>)
  n141 = local write "Output enabled"(w113) -> ()
  n142 = local write "Zoom freq X"(w113) -> ()
  n143 = local write "Zoom time Y"(w113) -> ()
  n144 = local write "Zoom time X"(w113) -> ()
  n145 = local write "Zoom freq Y"(w113) -> ()
  n146 = local write "freqdata"(cluster{"f0":dbl, "df":dbl, "magnitude":dbl[]}[] [] ("freqdata")) -> ()
  n147 = property on="Tab Control" class="TabCtl (strict)"() -> ("Pages"=w32:refnum<vi>[])  [unwired: 2 in, 2 out]
  n148 = property on="Setpoint enabled" class="Bool (strict)"("Val(Sgnl)"=FALSE ("Value (Signaling)")) -> ()  [unwired: 2 in, 2 out]
  n149 = Bundle By Name(cluster="Graph_refs", "upper.Graph"=w129, "upper.Time btn"=w128, "upper.Amplitude btn"=w127, "upper.Chart"=w126, "lower.Graph"=w125, "lower.Time btn"=w124, "lower.Amplitude btn"=w123, "lower.Chart"=w122, "Freq graph"=w121, "Adaptive FF graph"=w100) -> (w61:T15)
  n150 = property on="Unwrap phase" class="Bool (strict)"("Val(Sgnl)"=TRUE ("Value (Signaling)")) -> ()  [unwired: 2 in, 2 out]
  n151 = flat-sequence {
    tunnel: [w190] -> w33
    frame #0 {
      w190 = FALSE
      w191 = fxp<+/-,32,6> 0.0 ("Kp")
      n152 = local write "Enable"(w190) -> ()
      n153 = local write "Calculate w12"(w190) -> ()
      n154 = property on="Hold plot lower" class="Bool (strict)"("Value"=w190) -> ()  [unwired: 2 in, 2 out]
      n155 = local write "Kp Q"(w191) -> ()
      n156 = local write "Kd/T  Q"(w191) -> ()
      n157 = local write "Ki*T Q"(w191) -> ()
      n158 = local write "Kp AM"(w191) -> ()
      n159 = local write "Ki*T AM"(w191) -> ()
      n160 = local write "Kd/T AM"(w191) -> ()
    }
  }
  n161 = for {
    tunnel: w32 -> [w197] mode=indexing
    tunnel: w16 -> [w192]
    n162 = case shown="True" w192 {
      tunnel: ["Quench" ("y") "Cavity model" ("y")] -> w195
      frame False {
      }
      frame True {
      }
    }
    n163 = property class="Page"(reference=w197) -> (reference out=w194:refnum<vi>, "PageLabel"=w196:string)  [unwired: 1 in, 1 out]
    n164 = Not Equal?(x=w196, y=w195) -> (x != y?=w193:bool)
    n165 = property class="Page"(reference=w194, "PageVis"=w193) -> ()  [unwired: 1 in, 2 out]
  }
  n166 = Current VI's Path() -> (path=w60:path)
  n167 = register-events(w118) -> (reference out=w135:refnum<event-registration>)  [unwired: 2 in, 1 out]
  n168 = Bundle By Name(cluster=w69, "Vfi Vfq LP filter cut off frequency"=w3, "Vi Vq LP  filter cutoff fequency"=w4, "ch3 delay"=w5, "ch1 delay"=w6, "dw LP filter cut off frequency"=w7, "w12 LP  filter cutoff fequency"=w8, "dw scale"=w9, "w12 scale"=w10, "w12 - dt"=w11, "w12 - a"=w12, "w12 - b"=w13, "Mode"=w68, "Trigger"=w67, "Output mixer fequency [MHz]"=w66, "Output delay"=w65, "Mixer freq [MHz]"=w64, "Triggered"=w63, "Tranfer speed"=w46, "Continuous"=w62, "Output scale"=w53, "Host scale"=w51, "Input scale"=w50, "Host scale 5761"=w49, "Input scale 5761"=w48, "Virtual cavity"=w47, "Count to skip 5782, stage 1"=w43, "Count to skip 5761, stage 1"=w42, "K2"=w41, "Q2"=w40, "w2"=w39, "K3"=w38, "Q3"=w37, "w3"=w36, "w0"=w35, "Piezo"=w34, "Measure Tau at Time"=w31, "Tau set"=w30, "Count to skip 5761, stage 2"=w29, "Count to skip 5761, stage 3"=w28, "Count to skip 5782, stage 2"=w27, "Count to skip 5782, stage 3"=w26, "b"=w19, "a"=w18, "Fequency [kHz]"=w17) -> (w55:T3)
  "All FP controls" <- w55
  n169 = Open VI Reference(vi path=w60) -> (vi reference=w59:refnum<vi>)  [unwired: 5 in, 1 out]
  n170 = call "Init.vi"("vi reference"=w59, "Graph_refs"=w61, "SettingsFile in"=refnum<class "SettingsFileIQpid.lvclass"> refnum ("SettingsFileIQpid.lvclass")) -> ("Save event"=w57:T24, "SettingsFile out"=w56:refnum<class "SettingsFileIQpid.lvclass">)  [unwired: 6 in, 1 out]
  n171 = property on="Hold plot upper" class="Bool (strict)"("Val(Sgnl)"=w33) -> ()  [unwired: 2 in, 2 out]
  n172 = call "Init_IQ_PID.vi"("All FP controls"=w55, "SettingsFileIQpid in"=w56) -> ("SettingsFileIQpid out"=w14:refnum<class "SettingsFileIQpid.lvclass">)  [unwired: 8 in, 1 out]
  n173 = local write "Samples per 5782 record"(w112) -> ()
  n174 = local write "Mode"(w107) -> ()
  n175 = local write "Trigger"(w106) -> ()
  n176 = property class="VI"() -> ("Panel"=w45:refnum<vi>)  [unwired: 2 in, 2 out]
  n177 = control-ref of="Update once lower"() -> (w24:refnum<vi>)
  n178 = control-ref of="Update once upper"() -> (w25:refnum<vi>)
  n179 = case shown="No Error" w52 {
    tunnel: w101 -> [w212 w883]
    tunnel: [w211 w883] -> w103
    tunnel: w135 -> [w210 w882]
    tunnel: [w209 w882] -> w134
    tunnel: w61 -> [w207 _]
    tunnel: w112 -> [w206 _]
    tunnel: w57 -> [w205 _]
    tunnel: w45 -> [w204 w881]
    tunnel: [w203 w881] -> w44
    tunnel: w1 -> [w202 _]
    tunnel: w25 -> [w201 _]
    tunnel: w24 -> [w200 _]
    frame No Error {
      n180 = while {
        shift-right: [w221] -> w211
        shift-left: w212 -> [w228]
        tunnel: w210 -> [w226]
        tunnel: [w225] -> w209
        tunnel: [w224] -> w208
        tunnel: w207 -> [w223]
        tunnel: w206 -> [w222]
        tunnel: w205 -> [w219]
        shift-right: [w216] -> w203
        shift-left: w204 -> [w217]
        tunnel: w202 -> [w215]
        tunnel: w201 -> [w214]
        tunnel: w200 -> [w213]
        stop <- w224 stop-if-true
        n181 = call "GetTimeout.vi"("ScopeBase in"=w228) -> ("Time left"=w218:i32, "ScopeBase out"=w227:refnum<class "Scope5782_six_channel.lvclass">)  [unwired: 8 in, 1 out]
        n182 = event shown="[45] \"Output gain dB\": Value Change" {
          selector: w226 -> [_ _ _ _ _ _ _ _ _ _ _ _ _ _ _ _ _ _ _ _ _ _ _ _ _ _ _ _ _ _ _ _ _ _ _ _ _ _ _ _ _ _ _ _ _ _ _ _ _ _ _ _ _ _ _ _ _ _ _ _ _ _ _]
          dyn-events: [_ _ _ _ _ _ _ _ _ _ _ _ _ _ _ _ _ _ _ _ _ _ _ _ _ _ _ _ _ _ _ _ _ _ _ _ _ _ _ _ _ _ _ _ _ _ _ _ _ _ _ _ _ _ _ _ _ _ _ _ _ _ _] -> w225
          timeout: w218 -> [_ _ _ _ _ _ _ _ _ _ _ _ _ _ _ _ _ _ _ _ _ _ _ _ _ _ _ _ _ _ _ _ _ _ _ _ _ _ _ _ _ _ _ _ _ _ _ _ _ _ _ _ _ _ _ _ _ _ _ _ _ _ _]
          tunnel: [_ w286 _ _ _ _ _ _ _ _ _ _ _ _ _ _ _ _ _ _ _ _ _ _ _ _ _ _ _ _ _ _ "stop" _ _ _ _ _ _ _ _ _ _ _ _ _ _ _ _ _ _ _ _ _ _ _ _ _ _ _ _ _ _] -> w224
          tunnel: w227 -> [w255 w288 w299 w314 w317 w324 w334 w359 w379 w407 w413 w427 w433 w439 w445 w451 w457 w466 w470 w475 w488 w504 w506 w518 w528 w535 w540 w552 w582 w584 w590 w600 w602 w610 w622 w628 w636 w648 w656 w662 w672 w684 w690 w702 w708 w717 w723 w727 w734 w741 w743 w750 w756 w762 w769 w788 w794 w815 w828 w837 w844 w847 w877]
          tunnel: [w244 w288 w299 w312 w316 w321 w333 w358 w378 w406 w411 w423 w432 w438 w444 w450 w456 w460 w469 w476 w489 w503 w507 w517 w527 w533 w538 w546 w580 w585 w588 w600 w602 w610 w622 w628 w636 w648 w652 w660 w671 w683 w689 w701 w707 w717 w722 w726 w733 w740 w742 w749 w755 w761 w768 w786 w792 w801 w827 w834 w843 w846 w876] -> w221
          tunnel: w223 -> [_ _ _ _ _ _ _ _ _ _ _ _ _ _ _ _ _ _ _ _ _ _ _ _ _ _ _ _ _ _ _ _ _ _ _ _ _ w646 _ _ _ _ _ _ _ _ _ _ _ _ _ _ _ _ _ _ _ _ _ _ _ _ _]
          tunnel: w222 -> [_ _ _ _ _ _ _ _ _ _ _ _ _ _ _ _ _ _ _ _ _ _ _ _ _ _ _ w549 _ _ _ _ _ _ _ _ _ _ _ _ _ _ _ _ _ _ _ _ _ _ _ _ _ _ _ _ _ _ _ _ _ _ _]
          tunnel: w219 -> [_ w285 _ _ _ _ _ _ _ _ _ _ _ _ _ _ _ _ _ _ _ _ _ _ _ _ _ _ _ _ _ _ _ _ _ _ _ _ _ _ _ _ _ _ _ _ _ _ _ _ _ _ _ _ _ _ _ _ _ _ _ _ _]
          tunnel: [TRUE _ _ _ _ _ _ _ _ _ _ _ _ _ _ _ _ _ _ _ _ _ _ _ _ _ _ _ _ _ _ _ _ _ _ _ _ _ _ _ _ _ _ _ _ _ _ _ _ _ _ _ _ _ _ _ _ _ _ _ _ _ _] -> w220
          tunnel: [w232 w284 w295 w311 w315 w320 w339 w350 w370 w405 w422 w428 w429 w435 w441 w447 w453 w459 w468 w473 w486 w499 w505 w514 w523 w532 w537 w544 w579 w583 w589 w598 w601 w604 w614 w623 w629 w640 w651 w659 w667 w679 w685 w697 w703 w716 w718 w724 w730 w736 w747 w753 w759 w765 w783 w789 w799 w824 w833 w838 w845 w869 w880] -> w216
          tunnel: w217 -> [w242 w284 w295 w311 w315 w320 w339 w350 w370 w405 w422 w428 w429 w435 w441 w447 w453 w459 w468 w473 w486 w499 w505 w514 w523 w532 w537 w544 w579 w583 w589 w598 w601 w604 w614 w623 w629 w640 w651 w659 w667 w679 w685 w697 w703 w716 w718 w724 w730 w736 w747 w753 w759 w765 w783 w789 w799 w824 w833 w838 w845 w869 w880]
          tunnel: w215 -> [w256 _ _ _ _ _ _ _ _ _ _ _ _ _ _ _ _ _ _ _ _ _ _ _ _ _ _ _ _ _ _ _ _ _ _ _ _ _ _ _ _ _ _ _ _ w712 _ _ _ _ _ _ _ _ _ _ _ _ _ _ _ _ _]
          tunnel: w214 -> [w253 _ _ _ _ _ _ _ _ _ _ _ _ _ _ _ _ _ _ _ _ _ _ _ _ _ _ _ _ _ _ _ _ _ _ _ _ _ _ _ _ _ _ _ _ _ _ _ _ _ _ _ _ _ _ _ _ _ _ _ _ _ _]
          tunnel: w213 -> [w254 _ _ _ _ _ _ _ _ _ _ _ _ _ _ _ _ _ _ _ _ _ _ _ _ _ _ _ _ _ _ _ _ _ _ _ _ _ _ _ _ _ _ _ _ _ _ _ _ _ _ _ _ _ _ _ _ _ _ _ _ _ _]
          event Timeout {
            n183 = event-data() -> ()  [unwired: 1 in, 3 out]
            n184 = local read "Reference for phase"() -> (w252:T14)
            n185 = local read "Transfer speed"() -> (w250:T2)
            n186 = local read "Unwrap phase"() -> (w248:bool)
            n187 = property class="Pnl"(reference=w242, "DeferPanUpdts"=TRUE ("Defer Panel Updates")) -> (reference out=w235:refnum<vi>)  [unwired: 1 in, 1 out]
            n188 = local read "Window"() -> (w247:T13)
            n189 = local read "Display"() -> (w246:T18)
            n190 = local read "Buffer"() -> (w245:T17)
            n191 = local read "#bins"() -> (w251:i32)
            n192 = local read "Unit"() -> (w249:T12)
            n193 = call "AddDataToPlots.vi"("Scope5761 in"=w255, "Display"=w246, "Buffer"=w245, "Unwrap phase"=w248, "Transfer speed"=w250, "Reference for phase"=w252, "Window"=w247, "Unit"=w249, "#bins"=w251, "Update once lower"=w254, "Update once upper"=w253) -> ("Uppder data"=w239:dbl[][], "Lower data"=w237:dbl[][], "Scope5761 out"=w244:refnum<class "Scope5782_six_channel.lvclass">, "Freqdata"=w236:cluster{"f0":dbl, "df":dbl, "magnitude":dbl[]}[], "Any read?"=w243:bool, "Write upper"=w240:T29, "Write lower"=w238:T29)  [unwired: 10 in]
            n194 = local read "quench"() -> (w231:bool)
            n195 = case shown="\"Graph\"" w240 {
              selector: w240 -> [_ _ w283]
              tunnel: w239 -> [w281 w282 _]
              tunnel: [_ _ w283] -> w233
              frame "Graph" {
                "Upper graph" <- w281
              }
              frame "Chart" {
                "Upper chart" <- w282
              }
              frame "None", Default {
              }
            }
            n196 = case shown="\"Chart\"" w238 {
              selector: w238 -> [w277 _ _ _]
              tunnel: w237 -> [_ w278 w279 _]
              tunnel: w236 -> [_ _ _ w280]
              tunnel: [w277 _ _ _] -> w234
              frame "None", Default {
              }
              frame "Graph" {
                "Lower graph" <- w278
              }
              frame "Chart" {
                "Lower chart" <- w279
              }
              frame "Freq" {
                "freqdata" <- w280
              }
            }
            n197 = case shown="True" w231 {
              tunnel: w256 -> [_ w259]
              tunnel: w243 -> [_ w258]
              frame False {
              }
              frame True {
                n198 = case shown="True" w258 {
                  tunnel: w259 -> [_ w269]
                  frame False {
                  }
                  frame True {
                    n199 = xnode "Read/Write Control"("FPGA VI Reference In"=w269) -> ("FPGA VI Reference Out"=w261:refnum<k20>, "Quench_Warning"=w264:bool, "Amp1"=→"Amp1":fxp<+,16,14>, "TaM"=w267:fxp<+/-,32,13>, "Tau_set"=→"Tau_set":fxp<+/-,32,13>)  [unwired: 1 in, 1 out]
                    "Quench_Warning" <- w264
                    n200 = local read "Reset Quench Warning"() -> (w265:bool)
                    n201 = Compound Arithmetic op=AND(w265, invert w264) -> (w263:bool)
                    n202 = case shown="True" w263 {
                      tunnel: w261 -> [_ w273]
                      frame False {
                      }
                      frame True {
                        n203 = local write "Reset Quench Warning"(FALSE ("Reset Quench Warning")) -> ()
                        n204 = call "Write 16bit value.vi"("value"=fxp<+,16,16> 0.0, "FPGA Setting"=fpga_settings."Quench reset", "FPGA ref"=w273) -> ()  [unwired: 7 in, 2 out]
                      }
                    }
                    n205 = Multiply(x=w267, y=fxp<+/-,32,13> 6.399999618530273 ("x")) -> (x*y=→"Tau [µs]":fxp<+/-,64,26>)
                  }
                }
              }
            }
            n206 = flat-sequence {
              tunnel: w235 -> [w275]
              tunnel: w234 -> [_]
              tunnel: w233 -> [_]
              tunnel: [w274] -> w232
              frame #0 {
                n207 = property class="Pnl"(reference=w275, "DeferPanUpdts"=FALSE ("Defer Panel Updates")) -> (reference out=w274:refnum<vi>)  [unwired: 1 in, 1 out]
              }
            }
          }
          event Menu Selection (User) {
            n208 = event-data() -> ("ItemTag"=w287:string)  [unwired: 1 in, 6 out]
            n209 = case shown="\"Quit\"" w287 {
              tunnel: [_ w289 _ _] -> w286
              tunnel: w285 -> [_ _ w292 w294]
              frame "False", Default {
              }
              frame "Quit" {
                n210 = Two Button Dialog(message="Exit application?") -> (T button?=w289:bool)  [unwired: 2 in]
              }
              frame "SaveSettings" {
                n211 = Generate User Event(user event=w292, event data cluster=T25 {"Automatic"=FALSE, "Save"=TRUE} ("event data")) -> ()  [unwired: 2 in, 2 out]
              }
              frame "LoadSettings" {
                n212 = Generate User Event(user event=w294, event data cluster=T25 {"Automatic"=FALSE, "Save"=FALSE} ("event data")) -> ()  [unwired: 2 in, 2 out]
              }
            }
          }
          event Value Change {
            n213 = event-data() -> ("OldVal"=w296:T14)  [unwired: 1 in, 5 out]
            n214 = local read "Display"() -> (w297:T18)
            n215 = case shown="\"Phase and Magnitude\"" w297 {
              tunnel: "Reference for phase" -> [_ w304]
              tunnel: w296 -> [_ w302]
              frame "Time and Frequency", Default {
              }
              frame "Phase and Magnitude" {
                n216 = property on="Lower chart" class="WFChart (strict)"() -> ("History Data"=w303:dbl[][])  [unwired: 2 in, 2 out]
                n217 = Index Array(array=w303, index (row)=w302) -> (element=w301:dbl[])  [unwired: 1 in]
                n218 = Index Array(array=w303, index (row)=w304) -> (element=w305:dbl[])  [unwired: 1 in]
                n219 = for {
                  tunnel: w303 -> [w308] mode=indexing
                  tunnel: w305 -> [w310]
                  tunnel: [w309] -> w300 mode=indexing
                  tunnel: w301 -> [w307] mode=indexing
                  n220 = Add(x=w308, y=w307) -> (x+y=w306:dbl[])
                  n221 = Subtract(x=w306, y=w310) -> (x-y=w309:dbl[])
                }
                n222 = property on="Lower chart" class="WFChart (strict)"("History Data"=w300) -> ()  [unwired: 2 in, 2 out]
              }
            }
          }
          event "Mixer freq [MHz]": Value Change {
            n223 = event-data() -> ()  [unwired: 1 in, 6 out]
            n224 = call-dynamic "SetMixerFrequency.vi"("Mixer freq [MHz]"="Mixer freq [MHz]", "Scope5785_six_channel"=w314) -> ("Scope5785_six_channel Out"=w312:refnum<class "Scope5782_six_channel.lvclass">)  [unwired: 8 in, 1 out]
          }
          event "Fequency [MHz]", "Phase offset (deg)": Value Change {
            n225 = event-data() -> ()  [unwired: 1 in, 6 out]
            n226 = call-dynamic "SetSimulatedFreq.vi"("Phase offset (deg)"="Phase offset (deg)", "Mixer freq [MHz]"="Fequency [MHz]", "Scope5785_six_channel"=w317) -> ("Scope5785_six_channel out"=w316:refnum<class "Scope5782_six_channel.lvclass">)  [unwired: 7 in, 1 out]
          }
          event "Output mixer fequency [MHz]", "Output enabled": Value Change {
            n227 = event-data() -> ()  [unwired: 1 in, 6 out]
            n228 = call "SetOutputFreq.vi"("Output enabled"="Output enabled", "Output mixer fequency [MHz]"="Output mixer fequency [MHz]", "Scope5785_six_channel"=w324) -> ("Scope5785_six_channel out"=w321:refnum<class "Scope5782_six_channel.lvclass">)  [unwired: 7 in, 1 out]
          }
          event "Output delay", "Output delay delta": Value Change {
            w336 = fxp<+/-,16,2> 0.0 ("x")
            n229 = event-data() -> ()  [unwired: 1 in, 6 out]
            n230 = local read "Mixer freq [MHz]"() -> (w342:dbl)
            n231 = Multiply(x="Output delay", y=0.001) -> (x*y=w343:dbl)
            n232 = Multiply(x="Output delay delta", y=1e-06) -> (x*y=w345:dbl)
            n233 = call "Read FpgaRef5782.vi"("Scope5785_six_channel"=w334) -> ("FpgaRef5782.lvclass"=w332:refnum<class "FpgaRefx410.lvclass">, "Scope5785_six_channel Out"=w333:refnum<class "Scope5782_six_channel.lvclass">)  [unwired: 8 in, 1 out]
            n234 = Multiply(x=w342, y=6.283185307179586) -> (x*y=w340:dbl)
            n235 = Multiply(x=w340, y=w345) -> ()  [unwired: 1 out]
            n236 = Multiply(x=w343, y=w340) -> (x*y=w331:dbl)
            n237 = Sine & Cosine(0:w331) -> (1:w337:dbl, 2:w335:dbl)
            n238 = To Fixed-Point(fixed-point type=w336, number=w337) -> (fixed-point=w338:fxp<+/-,16,2>)
            n239 = To Fixed-Point(fixed-point type=w336, number=w335) -> (fixed-point=w330:fxp<+/-,16,2>)
            n240 = xnode "Reinterpret Number"("x"=w338) -> ("y"=w329:fxp<+,16,16>)
            n241 = xnode "Reinterpret Number"("x"=w330) -> ("y"=w328:fxp<+,16,16>)
            n242 = call "WriteSetting 16bit.vi"("value"=w329, "FPGA Setting"=fpga_settings."fixed sin_fi", "FpgaRefBase in"=w332) -> ("FpgaRefBase out"=w327:refnum<class "FpgaRefx410.lvclass">)  [unwired: 7 in, 1 out]
            n243 = call "WriteSetting 16bit.vi"("value"=w328, "FPGA Setting"=fpga_settings."fixed cos_fi", "FpgaRefBase in"=w327) -> ()  [unwired: 7 in, 2 out]
          }
          event "Ki*T AM", "Kd/T AM", "Kp AM": Value Change {
            n244 = event-data() -> ()  [unwired: 1 in, 6 out]
            n245 = xnode "Reinterpret Number"("x"="Kd/T AM") -> ("y"=w367:fxp<+,32,32>)
            n246 = xnode "Reinterpret Number"("x"="Ki*T AM") -> ("y"=w366:fxp<+,32,32>)
            n247 = xnode "Reinterpret Number"("x"="Kp AM") -> ("y"=w368:fxp<+,32,32>)
            n248 = To Unsigned Long Integer(number=w366) -> (unsigned 32bit integer=w353:u32)
            n249 = To Unsigned Long Integer(number=w367) -> (unsigned 32bit integer=w352:u32)
            n250 = To Unsigned Long Integer(number=w368) -> (unsigned 32bit integer=w351:u32)
            n251 = call "Write Setting 16bit.vi"("value"="I Feedback", "FPGA Setting"=fpga_settings."PID enabled I", "ScopeBase in"=w359) -> ("ScopeBase out"=w362:refnum<class "Scope5782_six_channel.lvclass">)  [unwired: 7 in, 1 out]
            n252 = call "Write Setting 32bit.vi"("value"=w353, "FPGA Setting"=fpga_settings."Ki*Tau am", "ScopeBase in"=w362) -> ("ScopeBase out"=w361:refnum<class "Scope5782_six_channel.lvclass">)  [unwired: 7 in, 1 out]
            n253 = call "Write Setting 32bit.vi"("value"=w352, "FPGA Setting"=fpga_settings."Kd_Tau am", "ScopeBase in"=w361) -> ("ScopeBase out"=w360:refnum<class "Scope5782_six_channel.lvclass">)  [unwired: 7 in, 1 out]
            n254 = call "Write Setting 32bit.vi"("value"=w351, "FPGA Setting"=fpga_settings."Kp am", "ScopeBase in"=w360) -> ("ScopeBase out"=w358:refnum<class "Scope5782_six_channel.lvclass">)  [unwired: 7 in, 1 out]
          }
          event "Kp Q", "Kd/T  Q", "Ki*T Q": Value Change {
            n255 = event-data() -> ()  [unwired: 1 in, 6 out]
            n256 = xnode "Reinterpret Number"("x"="Kd/T  Q") -> ("y"=w387:fxp<+,32,32>)
            n257 = xnode "Reinterpret Number"("x"="Ki*T Q") -> ("y"=w386:fxp<+,32,32>)
            n258 = xnode "Reinterpret Number"("x"="Kp Q") -> ("y"=w388:fxp<+,32,32>)
            n259 = To Unsigned Long Integer(number=w386) -> (unsigned 32bit integer=w373:u32)
            n260 = To Unsigned Long Integer(number=w387) -> (unsigned 32bit integer=w372:u32)
            n261 = To Unsigned Long Integer(number=w388) -> (unsigned 32bit integer=w371:u32)
            n262 = call "Write Setting 16bit.vi"("value"="Q Feedback", "FPGA Setting"=fpga_settings."Feedback Enable", "ScopeBase in"=w379) -> ("ScopeBase out"=w382:refnum<class "Scope5782_six_channel.lvclass">)  [unwired: 7 in, 1 out]
            n263 = call "Write Setting 32bit.vi"("value"=w373, "FPGA Setting"=fpga_settings."Ki*Tau Q", "ScopeBase in"=w382) -> ("ScopeBase out"=w381:refnum<class "Scope5782_six_channel.lvclass">)  [unwired: 7 in, 1 out]
            n264 = call "Write Setting 32bit.vi"("value"=w372, "FPGA Setting"=fpga_settings."Kd_Tau Q", "ScopeBase in"=w381) -> ("ScopeBase out"=w380:refnum<class "Scope5782_six_channel.lvclass">)  [unwired: 7 in, 1 out]
            n265 = call "Write Setting 32bit.vi"("value"=w371, "FPGA Setting"=fpga_settings."Kp Q", "ScopeBase in"=w380) -> ("ScopeBase out"=w378:refnum<class "Scope5782_six_channel.lvclass">)  [unwired: 7 in, 1 out]
          }
          event "w12", "R1", "w1", "Q1", "K1", "S", "K2", "Q2", "w2", "K3", "Q3", "w3": Value Change {
            n266 = event-data() -> ()  [unwired: 1 in, 6 out]
            n267 = call "CavityConstanstToFIFO.vi"("w12"="w12", "Mechanical mode"=1, "R1"="R1", "w1"="w1", "Q1"="Q1", "K1"="K1", "S"="S") -> ("FIFO array"=w404:u64[])  [unwired: 8 in]
            n268 = call "CavityConstanstToFIFO.vi"("w12"="w12", "Mechanical mode"=2, "R1"="R1", "w1"="w2", "Q1"="Q2", "K1"="K2", "S"="S") -> ("FIFO array"=w402:u64[])  [unwired: 8 in]
            n269 = call "CavityConstanstToFIFO.vi"("w12"="w12", "Mechanical mode"=3, "R1"="R1", "w1"="w3", "Q1"="Q3", "K1"="K3", "S"="S") -> ("FIFO array"=w389:u64[])  [unwired: 8 in]
            n270 = Build Array (concatenate)(w404, w402, w389) -> (w403:u64[])
            n271 = call "Write Setting Array.vi"("Data"=w403, "ScopeBase in"=w407) -> ("ScopeBase out"=w406:refnum<class "Scope5782_six_channel.lvclass">)  [unwired: 8 in, 1 out]
          }
          event "w0": Value Change {
            w416 = 1e-07  # dt
            n272 = event-data() -> ()  [unwired: 1 in, 6 out]
            n273 = Multiply(x="w0", y=w416) -> (x*y=w415:dbl)
            n274 = To Fixed-Point(fixed-point type=fxp<+/-,48,0> 0.0 ("x"), number=w415) -> (fixed-point=w421:fxp<+/-,48,0>)
            n275 = xnode "Reinterpret Number"("x"=w421) -> ("y"=w419:fxp<+,48,48>)
            n276 = call "To48BitSetting.vi"("48 bit value"=w419, "FPGA Setting"=fpga_settings."Cavity_w0_dt") -> ("value"=w414:u64)  [unwired: 9 in]
            n277 = Build Array(w414) -> (w412:u64[])
            n278 = call "Write Setting Array.vi"("Data"=w412, "ScopeBase in"=w413) -> ("ScopeBase out"=w411:refnum<class "Scope5782_six_channel.lvclass">)  [unwired: 8 in, 1 out]
          }
          event Value Change {
            n279 = event-data() -> ()  [unwired: 1 in, 6 out]
            n280 = To Unsigned Long Integer(number="Piezo") -> (unsigned 32bit integer=w424:u32)
            n281 = call "Write Setting 32bit.vi"("value"=w424, "FPGA Setting"=fpga_settings."Piezo setting", "ScopeBase in"=w427) -> ("ScopeBase out"=w423:refnum<class "Scope5782_six_channel.lvclass">)  [unwired: 7 in, 1 out]
          }
          event "ch0 DC offset": Value Change {
            n282 = event-data() -> ()  [unwired: 1 in, 6 out]
            n283 = call "Read FpgaRef5782.vi"("Scope5785_six_channel"=w433) -> ("FpgaRef5782.lvclass"=w434:refnum<class "FpgaRefx410.lvclass">, "Scope5785_six_channel Out"=w432:refnum<class "Scope5782_six_channel.lvclass">)  [unwired: 8 in, 1 out]
            n284 = call "SetDcOffset.vi"("FPGA Setting"=fpga_settings."DC_offs 0", "DC offset"="ch0 DC offset", "FpgaRef5782 in"=w434) -> ()  [unwired: 7 in, 2 out]
          }
          event "ch0 DC offset 2": Value Change {
            n285 = event-data() -> ()  [unwired: 1 in, 6 out]
            n286 = call "Read FpgaRef5761.vi"("Scope5785_six_channel"=w439) -> ("FpgaRef5761.lvclass"=w440:refnum<class "FpgaRef5761.lvclass">, "Scope5785_six_channel Out"=w438:refnum<class "Scope5782_six_channel.lvclass">)  [unwired: 8 in, 1 out]
            n287 = call "SetDcOffset.vi"("FPGA Setting"=fpga_settings."DC_offs 0", "DC offset"="ch0 DC offset 2", "FpgaRef5761 In"=w440) -> ()  [unwired: 7 in, 2 out]
          }
          event "ch1 DC offset 2": Value Change {
            n288 = event-data() -> ()  [unwired: 1 in, 6 out]
            n289 = call "Read FpgaRef5761.vi"("Scope5785_six_channel"=w445) -> ("FpgaRef5761.lvclass"=w446:refnum<class "FpgaRef5761.lvclass">, "Scope5785_six_channel Out"=w444:refnum<class "Scope5782_six_channel.lvclass">)  [unwired: 8 in, 1 out]
            n290 = call "SetDcOffset.vi"("FPGA Setting"=fpga_settings."DC_offs 1", "DC offset"="ch1 DC offset 2", "FpgaRef5761 In"=w446) -> ()  [unwired: 7 in, 2 out]
          }
          event "ch2 DC offset": Value Change {
            n291 = event-data() -> ()  [unwired: 1 in, 6 out]
            n292 = call "Read FpgaRef5761.vi"("Scope5785_six_channel"=w451) -> ("FpgaRef5761.lvclass"=w452:refnum<class "FpgaRef5761.lvclass">, "Scope5785_six_channel Out"=w450:refnum<class "Scope5782_six_channel.lvclass">)  [unwired: 8 in, 1 out]
            n293 = call "SetDcOffset.vi"("FPGA Setting"=fpga_settings."DC_offs 2", "DC offset"="ch2 DC offset", "FpgaRef5761 In"=w452) -> ()  [unwired: 7 in, 2 out]
          }
          event "ch3 DC offset": Value Change {
            n294 = event-data() -> ()  [unwired: 1 in, 6 out]
            n295 = call "Read FpgaRef5761.vi"("Scope5785_six_channel"=w457) -> ("FpgaRef5761.lvclass"=w458:refnum<class "FpgaRef5761.lvclass">, "Scope5785_six_channel Out"=w456:refnum<class "Scope5782_six_channel.lvclass">)  [unwired: 8 in, 1 out]
            n296 = call "SetDcOffset.vi"("FPGA Setting"=fpga_settings."DC_offs 3", "DC offset"="ch3 DC offset", "FpgaRef5761 In"=w458) -> ()  [unwired: 7 in, 2 out]
          }
          event "Feedback delay", "Trigger delay": Value Change {
            n297 = event-data() -> ()  [unwired: 1 in, 6 out]
            n298 = Add(x="Feedback delay", y="Trigger delay") -> (x+y=w464:u32)
            n299 = call "Write Setting 32bit.vi"("value"=w464, "FPGA Setting"=fpga_settings."Feedback delay", "ScopeBase in"=w466) -> ("ScopeBase out"=w462:refnum<class "Scope5782_six_channel.lvclass">)  [unwired: 7 in, 1 out]
            n300 = call "Write Setting 32bit.vi"("value"="Trigger delay", "FPGA Setting"=fpga_settings."Trigger delay", "ScopeBase in"=w462) -> ("ScopeBase out"=w460:refnum<class "Scope5782_six_channel.lvclass">)  [unwired: 7 in, 1 out]
          }
          event "Acquire samples": Value Change {
            n301 = event-data() -> ()  [unwired: 1 in, 6 out]
            n302 = call "Write Setting 32bit.vi"("value"="Acquire samples", "FPGA Setting"=fpga_settings."Samples to acquire", "ScopeBase in"=w470) -> ("ScopeBase out"=w469:refnum<class "Scope5782_six_channel.lvclass">)  [unwired: 7 in, 1 out]
          }
          event "show setpoint": Value Change {
            n303 = event-data() -> ()  [unwired: 1 in, 6 out]
            n304 = call "Read Feedforward.vi"("Scope5785_six_channel"=w475) -> ("Feeforward"=w474:T30, "Scope5785_six_channel out"=w476:refnum<class "Scope5782_six_channel.lvclass">)  [unwired: 8 in, 1 out]
            n305 = Unbundle By Name(w474) -> ("Setpoint I"=w483:dbl[], "Setpoint Q"=w482:dbl[])
            n306 = Array Size(array=w483) -> (size(s)=w481:i32)
            n307 = Array Size(array=w482) -> (size(s)=w480:i32)
            n308 = Build Array(w483, w482) -> (w484:dbl[][])
            n309 = Greater Than 0?(x=w481) -> (x > 0?=w479:bool)
            n310 = Greater Than 0?(x=w480) -> (x > 0?=w478:bool)
            n311 = And(x=w479, y=w478) -> (x .and. y?=w477:bool)
            n312 = case shown="True" w477 {
              tunnel: w484 -> [_ w485]
              frame False {
              }
              frame True {
                n313 = call "ShowIQvaluesAsync.vi"("IQ data"=w485) -> ()  [unwired: 11 in]
              }
            }
          }
          event "show feedforward": Value Change {
            n314 = event-data() -> ()  [unwired: 1 in, 6 out]
            n315 = call "Read Feedforward.vi"("Scope5785_six_channel"=w488) -> ("Feeforward"=w487:T30, "Scope5785_six_channel out"=w489:refnum<class "Scope5782_six_channel.lvclass">)  [unwired: 8 in, 1 out]
            n316 = Unbundle By Name(w487) -> ("Feedforward I"=w496:dbl[], "Feedforward Q"=w495:dbl[])
            n317 = Array Size(array=w496) -> (size(s)=w494:i32)
            n318 = Array Size(array=w495) -> (size(s)=w493:i32)
            n319 = Build Array(w496, w495) -> (w497:dbl[][])
            n320 = Greater Than 0?(x=w494) -> (x > 0?=w492:bool)
            n321 = Greater Than 0?(x=w493) -> (x > 0?=w491:bool)
            n322 = And(x=w492, y=w491) -> (x .and. y?=w490:bool)
            n323 = case shown="True" w490 {
              tunnel: w497 -> [_ w498]
              frame False {
              }
              frame True {
                n324 = call "ShowIQvaluesAsync.vi"("IQ data"=w498) -> ()  [unwired: 11 in]
              }
            }
          }
          event "ch1 DC offset": Value Change {
            n325 = event-data() -> ()  [unwired: 1 in, 6 out]
            n326 = call "Read FpgaRef5782.vi"("Scope5785_six_channel"=w504) -> ("FpgaRef5782.lvclass"=w502:refnum<class "FpgaRefx410.lvclass">, "Scope5785_six_channel Out"=w503:refnum<class "Scope5782_six_channel.lvclass">)  [unwired: 8 in, 1 out]
            n327 = call "SetDcOffset.vi"("FPGA Setting"=fpga_settings."DC_offs 1", "DC offset"="ch1 DC offset", "FpgaRef5782 in"=w502) -> ()  [unwired: 7 in, 2 out]
          }
          event "Setpoint enabled": Value Change {
            n328 = event-data() -> ()  [unwired: 1 in, 6 out]
            n329 = Boolean To (0,1)(Boolean="Setpoint enabled") -> (0, 1=w510:i16)
            n330 = To Word Integer(number=w510) -> (16bit integer=w512:i16)
            n331 = xnode "Reinterpret Number"("x"=w512) -> ("y"=w513:fxp<+/-,16,14>)
            n332 = xnode "Reinterpret Number"("x"=w513) -> ("y"=w509:fxp<+,16,16>)
            n333 = call "Write Setting 16bit.vi"("value"=w509, "FPGA Setting"=fpga_settings."Setpoint enable", "ScopeBase in"=w506) -> ("ScopeBase out"=w507:refnum<class "Scope5782_six_channel.lvclass">)  [unwired: 7 in, 1 out]
          }
          event "Cavity model": Value Change {
            n334 = event-data() -> ()  [unwired: 1 in, 6 out]
            n335 = Boolean To (0,1)(Boolean="Cavity model") -> (0, 1=w520:i16)
            n336 = To Word Integer(number=w520) -> (16bit integer=w521:i16)
            n337 = xnode "Reinterpret Number"("x"=w521) -> ("y"=w522:fxp<+/-,16,14>)
            n338 = xnode "Reinterpret Number"("x"=w522) -> ("y"=w515:fxp<+,16,16>)
            n339 = call "Write Setting 16bit.vi"("value"=w515, "FPGA Setting"=fpga_settings."Cavity Enable", "ScopeBase in"=w518) -> ("ScopeBase out"=w517:refnum<class "Scope5782_six_channel.lvclass">)  [unwired: 7 in, 1 out]
          }
          event "Virtual cavity": Value Change {
            n340 = event-data() -> ()  [unwired: 1 in, 6 out]
            n341 = Boolean To (0,1)(Boolean="Virtual cavity") -> (0, 1=w529:i16)
            n342 = To Word Integer(number=w529) -> (16bit integer=w530:i16)
            n343 = xnode "Reinterpret Number"("x"=w530) -> ("y"=w531:fxp<+/-,16,14>)
            n344 = xnode "Reinterpret Number"("x"=w531) -> ("y"=w525:fxp<+,16,16>)
            n345 = call "Write Setting 16bit.vi"("value"=w525, "FPGA Setting"=fpga_settings."Virtual cavity", "ScopeBase in"=w528) -> ("ScopeBase out"=w527:refnum<class "Scope5782_six_channel.lvclass">)  [unwired: 7 in, 1 out]
          }
          event Value Change {
            n346 = event-data() -> ()  [unwired: 1 in, 6 out]
            n347 = property on="Rumode" class="Bool (strict)"("Val(Sgnl)"=FALSE ("Value (Signaling)")) -> ()  [unwired: 2 in, 2 out]
            n348 = call-dynamic "SetMode.vi"("Mode"="Mode", "ScopeBase In"=w535) -> ("ScopeBase Out"=w533:refnum<class "Scope5782_six_channel.lvclass">)  [unwired: 8 in, 1 out]
          }
          event Value Change {
            n349 = event-data() -> ()  [unwired: 1 in, 6 out]
            n350 = call-dynamic "SetTrigger.vi"("Trigger"="Trigger", "ScopeBase In"=w540) -> ("ScopeBase Out"=w538:refnum<class "Scope5782_six_channel.lvclass">)  [unwired: 8 in, 1 out]
          }
          event Value Change {
            w554 = dbl[][] [] ("History Data")
            n351 = event-data() -> ()  [unwired: 1 in, 6 out]
            n352 = case shown="\"High speed (10Ms/s)\"" "Transfer speed" {
              tunnel: [w562 w568 w576] -> w548
              tunnel: w549 -> [w563 w571 w576]
              tunnel: [0.0001 ("t") 0.02 ("t") 0.001 ("t")] -> w550
              tunnel: [T27."Disabled and Grayed Out" ("Disabled") T27."Enabled" ("Disabled") T27."Disabled and Grayed Out" ("Disabled")] -> w543
              tunnel: [6 ("dimension size") 14 ("dimension size") 14 ("dimension size")] -> w541
              frame "High speed (10Ms/s)" {
                n353 = Multiply(x=10, y=w563) -> (x*y=w562:i32)
              }
              frame "Ultra low speed (50kS/s)" {
                n354 = Divide(x=w571, y=20 ("x")) -> (x/y=w570:dbl)
                n355 = Round To Nearest(number=w570) -> (nearest integer value=w569:dbl)
                n356 = To Long Integer(number=w569) -> (32bit integer=w568:i32)
              }
              frame "Low speed (1Ms/s)" {
              }
            }
            n357 = property on="FFT buffer size" class="Enum (strict)"("DisabledEnum"=w543) -> ()  [unwired: 2 in, 2 out]
            n358 = call-dynamic "SetRecordLength.vi"("Samples per 5782 record"=w548, "ScopeBase In"=w552) -> ("ScopeBase Out"=w551:refnum<class "Scope5782_six_channel.lvclass">)  [unwired: 8 in, 1 out]
            n359 = property on="Lower chart" class="WFChart (strict)"("History Data"=w554) -> ()  [unwired: 2 in, 2 out]
            n360 = property on="Upper chart" class="WFChart (strict)"("History Data"=w554) -> (error out=w555:errorcluster)  [unwired: 2 in, 1 out]
            n361 = Initialize Array(nan ("element"), 4 ("dimension size"), w548) -> (w557:dbl[][])
            n362 = call-dynamic "SetFullSpeedTransfer.vi"("Tranfer speed"="Transfer speed", "ScopeBase In"=w551) -> ("ScopeBase Out"=w547:refnum<class "Scope5782_six_channel.lvclass">)  [unwired: 8 in, 1 out]
            n363 = property on="Upper chart" class="WFChart (strict)"("XScale.Multiplier"=w550) -> ()  [unwired: 2 in, 2 out]
            n364 = flat-sequence {
              tunnel: w557 -> [w578]
              tunnel: [w577] -> w553
              tunnel: w555 -> [_]
              frame #0 {
                n365 = local write "Upper chart"(w578) -> ()
                n366 = local read "Zoom time X"() -> (w577:bool)
              }
            }
            n367 = call-dynamic "InitFFT_Buffer.vi"("FFT buffer size"="FFT buffer size", "dimension size"=w541, "Transfer speed"="Transfer speed", "ScopeBase In"=w547) -> ("ScopeBase Out"=w546:refnum<class "Scope5782_six_channel.lvclass">)  [unwired: 6 in, 1 out]
            n368 = property on="Zoom time X" class="Bool (strict)"("Val(Sgnl)"=w553) -> ()  [unwired: 2 in, 2 out]
          }
          event "Samples per 5782 record": Value Change {
            n369 = event-data() -> ()  [unwired: 1 in, 6 out]
            n370 = call-dynamic "SetRecordLength.vi"("Samples per 5782 record"="Samples per 5782 record", "ScopeBase In"=w582) -> ("ScopeBase Out"=w580:refnum<class "Scope5782_six_channel.lvclass">)  [unwired: 8 in, 1 out]
          }
          event "Singleshot": Value Change {
            n371 = event-data() -> ()  [unwired: 1 in, 6 out]
            n372 = local write "Rumode"(FALSE ("Rumode")) -> ()
            n373 = call-dynamic "SetRunMode.vi"("RunMode"=ScopeMode."Single" ("scope mode"), "ScopeBase in"=w584) -> ("ScopeBase out"=w585:refnum<class "Scope5782_six_channel.lvclass">)  [unwired: 8 in, 1 out]
          }
          event "Rumode": Value Change {
            n374 = event-data() -> ()  [unwired: 1 in, 6 out]
            n375 = case shown="\"Triggered\"" "Trigmode" {
              tunnel: [ScopeMode."Running" ("scope mode") ScopeMode."Continuous" ("scope mode")] -> w592
              frame "Triggered" {
              }
              frame "Continuous" {
              }
            }
            n376 = Select(t=w592, s="Rumode", f=ScopeMode."Stopped" ("scope mode")) -> (s? t:f=w591:T28)
            n377 = call-dynamic "SetRunMode.vi"("RunMode"=w591, "ScopeBase in"=w590) -> ("ScopeBase out"=w588:refnum<class "Scope5782_six_channel.lvclass">)  [unwired: 8 in, 1 out]
          }
          event "Unwrap phase": Value Change {
            w599 = dbl[][] [] ("History Data")
            n378 = event-data() -> ()  [unwired: 1 in, 6 out]
            n379 = property on="Lower chart" class="WFChart (strict)"("History Data"=w599) -> ()  [unwired: 2 in, 2 out]
            n380 = property on="Upper chart" class="WFChart (strict)"("History Data"=w599) -> ()  [unwired: 2 in, 2 out]
          }
          event "stop": Value Change {
            n381 = event-data() -> ()  [unwired: 1 in, 6 out]
          }
          event Value Change {
            n382 = event-data() -> ()  [unwired: 1 in, 6 out]
            n383 = case shown="\"V\"" "Unit" {
              tunnel: ["V" "dBV" "V^2"] -> w607
              frame "V" {
              }
              frame "dBV" {
              }
              frame "V^2" {
              }
            }
            n384 = Concatenate Strings("Amplitude [", w607, "]") -> (w605:string)
            n385 = property on="freqdata" class="WFGraph (strict)"("YScale.NameLbl.Text"=w605) -> ()  [unwired: 2 in, 2 out]
          }
          event "#bins": Value Change {
            n386 = event-data() -> ()  [unwired: 1 in, 6 out]
            n387 = local read "Upper chart"() -> (w618:dbl[][])
            n388 = local read "Window"() -> (w619:T13)
            n389 = local read "Unit"() -> (w620:T12)
            n390 = call "calc FFT_indexed.vi"("#bins"="#bins", "IQ indexes"=i32[][] [[0, 1], [2, 3], [4, 5], [6, 7], [8, 9], [10, 11], [12, 13]], "dt"=1e-06, "Unit"=w620, "Window"=w619, "data"=w618) -> ("Power Spectrum / PSD"=w617:cluster{"f0":dbl, "df":dbl, "magnitude":dbl[]}[])  [unwired: 5 in]
            n391 = local write "freqdata"(w617) -> ()
          }
          event "Zoom time X", "Zoom time Y": Value Change {
            n392 = event-data() -> ()  [unwired: 1 in, 6 out]
            n393 = control-ref of="Upper chart"() -> (w626:refnum<vi>)
            n394 = control-ref of="Upper graph"() -> (w627:refnum<vi>)
            n395 = call "setZoomTool.vi"("Zoom Y"="Zoom time Y", "Zoom  X"="Zoom time X", "reference"=w626) -> ()  [unwired: 9 in]
            n396 = call "setZoomTool.vi"("Zoom Y"="Zoom time Y", "Zoom  X"="Zoom time X", "reference"=w627) -> ()  [unwired: 9 in]
          }
          event "Zoom freq Y", "Zoom freq X": Value Change {
            n397 = event-data() -> ()  [unwired: 1 in, 6 out]
            n398 = control-ref of="Lower graph"() -> (w633:refnum<vi>)
            n399 = control-ref of="Lower chart"() -> (w634:refnum<vi>)
            n400 = control-ref of="Adaptive FF graph"() -> (w630:refnum<vi>)
            n401 = control-ref of="freqdata"() -> (w635:refnum<vi>)
            n402 = call "setZoomTool.vi"("Zoom Y"="Zoom freq Y", "Zoom  X"="Zoom freq X", "reference"=w635) -> ()  [unwired: 9 in]
            n403 = call "setZoomTool.vi"("Zoom Y"="Zoom freq Y", "Zoom  X"="Zoom freq X", "reference"=w630) -> ()  [unwired: 9 in]
            n404 = call "setZoomTool.vi"("Zoom Y"="Zoom freq Y", "Zoom  X"="Zoom freq X", "reference"=w634) -> ()  [unwired: 9 in]
            n405 = call "setZoomTool.vi"("Zoom Y"="Zoom freq Y", "Zoom  X"="Zoom freq X", "reference"=w633) -> ()  [unwired: 9 in]
          }
          event "Show buffers": Value Change {
            n406 = event-data() -> ("CtlRef"=w643:refnum<vi>)  [unwired: 1 in, 5 out]
            n407 = control-ref of="Show buffers"() -> (w642:refnum<vi>)
            n408 = Equal?(x=w643, y=w642) -> (x = y?=w641:bool)
            n409 = case shown="False" w641 {
              frame False {
                w649 = dbl[][] [] ("History Data")
                n410 = local write "freqdata"(cluster{"f0":dbl, "df":dbl, "magnitude":dbl[]}[] [] ("freqdata")) -> ()
                n411 = property on="Upper chart" class="WFChart (strict)"("History Data"=w649) -> ()  [unwired: 2 in, 2 out]
                n412 = local write "Lower graph"(w649) -> ()
                n413 = local write "Upper graph"(w649) -> ()
                n414 = property on="Lower chart" class="WFChart (strict)"("History Data"=w649) -> ()  [unwired: 2 in, 2 out]
              }
              frame True {
              }
            }
            n415 = local read "Transfer speed"() -> (w637:T2)
            n416 = call "UpdateGraphs.vi"("Transfer speed"=w637, "Show buffers"="Show buffers", "Buffer mode"="Buffer", "Display mode"="Display", "Graph_refs"=w646) -> ("Graph_refs out"=w639:T15)  [unwired: 6 in]
            n417 = call "UpdateGraphLegends.vi"("Display"="Display", "Graph_refs"=w639) -> ()  [unwired: 9 in, 1 out]
            n418 = property on="Zoom time X" class="Bool (strict)"("Val(Sgnl)"=TRUE ("Value (Signaling)")) -> ()  [unwired: 2 in, 2 out]
          }
          event "Feed forward": Value Change {
            n419 = event-data() -> ()  [unwired: 1 in, 6 out]
            n420 = control-ref of="show feedforward"() -> (w658:refnum<vi>)
            n421 = call "LoadFeedforward.vi"("show ref"=w658, "Path"="Feed forward") -> ("error out"=w653:errorcluster, "values Q"=w654:dbl[], "values I"=w655:dbl[])  [unwired: 7 in]
            n422 = call "SetFeedForward.vi"("error in (no error)"=w653, "values Q"=w654, "values I"=w655, "Scope5785_six_channel"=w656) -> ("Scope5785_six_channel out"=w652:refnum<class "Scope5782_six_channel.lvclass">)  [unwired: 6 in, 1 out]
          }
          event "Setpoint": Value Change {
            n423 = event-data() -> ()  [unwired: 1 in, 6 out]
            n424 = control-ref of="show setpoint"() -> (w666:refnum<vi>)
            n425 = call "LoadFeedforward.vi"("show ref"=w666, "Path"="Setpoint") -> ("error out"=w661:errorcluster, "values Q"=w663:dbl[], "values I"=w664:dbl[])  [unwired: 7 in]
            n426 = call "SetSetpoint.vi"("error in (no error)"=w661, "values Q"=w663, "values I"=w664, "Scope5785_six_channel"=w662) -> ("Scope5785_six_channel out"=w660:refnum<class "Scope5782_six_channel.lvclass">)  [unwired: 6 in, 1 out]
          }
          event "Input delay 5761": Value Change {
            n427 = event-data() -> ()  [unwired: 1 in, 6 out]
            n428 = call "Read FpgaRef5761.vi"("Scope5785_six_channel"=w672) -> ("FpgaRef5761.lvclass"=w670:refnum<class "FpgaRef5761.lvclass">, "Scope5785_six_channel Out"=w671:refnum<class "Scope5782_six_channel.lvclass">)  [unwired: 8 in, 1 out]
            n429 = call "WriteSetting 32bit.vi"("value"="Input delay 5761", "FPGA Setting"=fpga_settings."Input delay", "FpgaRefBase in"=w670) -> ()  [unwired: 7 in, 2 out]
          }
          event "Count to skip 5761, stage 1": Value Change {
            n430 = event-data() -> ()  [unwired: 1 in, 6 out]
            n431 = call "Read FpgaRef5761.vi"("Scope5785_six_channel"=w684) -> ("FpgaRef5761.lvclass"=w682:refnum<class "FpgaRef5761.lvclass">, "Scope5785_six_channel Out"=w683:refnum<class "Scope5782_six_channel.lvclass">)  [unwired: 8 in, 1 out]
            n432 = call "WriteSetting 32bit.vi"("value"="Count to skip 5761, stage 1", "FPGA Setting"=fpga_settings."Samples to skip", "FpgaRefBase in"=w682) -> ("FpgaRefBase out"=w673:refnum<class "FpgaRef5761.lvclass">)  [unwired: 7 in, 1 out]
            n433 = call "WriteSetting 32bit.vi"("value"="Count to skip 5761, stage 2", "FPGA Setting"=fpga_settings."Samples to skip 2", "FpgaRefBase in"=w673) -> ("FpgaRefBase out"=w678:refnum<class "FpgaRef5761.lvclass">)  [unwired: 7 in, 1 out]
            n434 = call "WriteSetting 32bit.vi"("value"="Count to skip 5761, stage 3", "FPGA Setting"=fpga_settings."Samples to skip 3", "FpgaRefBase in"=w678) -> ()  [unwired: 7 in, 2 out]
          }
          event "Input delay 5782": Value Change {
            n435 = event-data() -> ()  [unwired: 1 in, 6 out]
            n436 = call "Read FpgaRef5782.vi"("Scope5785_six_channel"=w690) -> ("FpgaRef5782.lvclass"=w688:refnum<class "FpgaRefx410.lvclass">, "Scope5785_six_channel Out"=w689:refnum<class "Scope5782_six_channel.lvclass">)  [unwired: 8 in, 1 out]
            n437 = call "WriteSetting 32bit.vi"("value"="Input delay 5782", "FPGA Setting"=fpga_settings."Input delay", "FpgaRefBase in"=w688) -> ()  [unwired: 7 in, 2 out]
          }
          event "Count to skip 5782, stage 1", "Count to skip 5782, stage 2", "Count to skip 5782, stage 3": Value Change {
            n438 = event-data() -> ()  [unwired: 1 in, 6 out]
            n439 = call "Read FpgaRef5782.vi"("Scope5785_six_channel"=w702) -> ("FpgaRef5782.lvclass"=w700:refnum<class "FpgaRefx410.lvclass">, "Scope5785_six_channel Out"=w701:refnum<class "Scope5782_six_channel.lvclass">)  [unwired: 8 in, 1 out]
            n440 = call "WriteSetting 32bit.vi"("value"="Count to skip 5782, stage 1", "FPGA Setting"=fpga_settings."Samples to skip", "FpgaRefBase in"=w700) -> ("FpgaRefBase out"=w692:refnum<class "FpgaRefx410.lvclass">)  [unwired: 7 in, 1 out]
            n441 = call "WriteSetting 32bit.vi"("value"="Count to skip 5782, stage 2", "FPGA Setting"=fpga_settings."Samples to skip 2", "FpgaRefBase in"=w692) -> ("FpgaRefBase out"=w693:refnum<class "FpgaRefx410.lvclass">)  [unwired: 7 in, 1 out]
            n442 = call "WriteSetting 32bit.vi"("value"="Count to skip 5782, stage 3", "FPGA Setting"=fpga_settings."Samples to skip 3", "FpgaRefBase in"=w693) -> ()  [unwired: 7 in, 2 out]
          }
          event Value Change {
            n443 = event-data() -> ()  [unwired: 1 in, 6 out]
            n444 = call "Read FpgaRef5782.vi"("Scope5785_six_channel"=w708) -> ("FpgaRef5782.lvclass"=w706:refnum<class "FpgaRefx410.lvclass">, "Scope5785_six_channel Out"=w707:refnum<class "Scope5782_six_channel.lvclass">)  [unwired: 8 in, 1 out]
            n445 = call "WriteSetting 16bit.vi"("value"="Output scale", "FPGA Setting"=fpga_settings."Output scale", "FpgaRefBase in"=w706) -> ()  [unwired: 7 in, 2 out]
          }
          event "Output gain dB": Value Change {
            n446 = event-data() -> ()  [unwired: 1 in, 6 out]
            n447 = Divide(x="Output gain dB", y=20.0) -> (x/y=w714:dbl)
            n448 = Power Of 10(x=w714) -> (10^x=w713:dbl)
            n449 = To Fixed-Point(fixed-point type=fxp<+/-,16,10> 0.0 ("Output gain"), number=w713) -> (fixed-point=w709:fxp<+/-,16,10>)
            n450 = xnode "Read/Write Control"("FPGA VI Reference In"=w712, "Output gain"=w709) -> ()  [unwired: 1 in, 2 out]
          }
          event Value Change {
            n451 = event-data() -> ()  [unwired: 1 in, 6 out]
            n452 = call "Read FpgaRef5782.vi"("Scope5785_six_channel"=w723) -> ("FpgaRef5782.lvclass"=w721:refnum<class "FpgaRefx410.lvclass">, "Scope5785_six_channel Out"=w722:refnum<class "Scope5782_six_channel.lvclass">)  [unwired: 8 in, 1 out]
            n453 = call "WriteSetting 16bit.vi"("value"="Input scale", "FPGA Setting"=fpga_settings."Input scale", "FpgaRefBase in"=w721) -> ()  [unwired: 7 in, 2 out]
          }
          event Value Change {
            n454 = event-data() -> ()  [unwired: 1 in, 6 out]
            n455 = call "Read FpgaRef5761.vi"("Scope5785_six_channel"=w727) -> ("FpgaRef5761.lvclass"=w725:refnum<class "FpgaRef5761.lvclass">, "Scope5785_six_channel Out"=w726:refnum<class "Scope5782_six_channel.lvclass">)  [unwired: 8 in, 1 out]
            n456 = call "WriteSetting 16bit.vi"("value"="Input scale 5761", "FPGA Setting"=fpga_settings."Input scale", "FpgaRefBase in"=w725) -> ()  [unwired: 7 in, 2 out]
          }
          event Value Change {
            n457 = event-data() -> ()  [unwired: 1 in, 6 out]
            n458 = call "Read FpgaRef5761.vi"("Scope5785_six_channel"=w734) -> ("FpgaRef5761.lvclass"=w732:refnum<class "FpgaRef5761.lvclass">, "Scope5785_six_channel Out"=w733:refnum<class "Scope5782_six_channel.lvclass">)  [unwired: 8 in, 1 out]
            n459 = call "WriteSetting 16bit.vi"("value"="Host scale 5761", "FPGA Setting"=fpga_settings."Host scale", "FpgaRefBase in"=w732) -> ()  [unwired: 7 in, 2 out]
          }
          event Value Change {
            n460 = event-data() -> ()  [unwired: 1 in, 6 out]
            n461 = call "Read FpgaRef5782.vi"("Scope5785_six_channel"=w741) -> ("FpgaRef5782.lvclass"=w739:refnum<class "FpgaRefx410.lvclass">, "Scope5785_six_channel Out"=w740:refnum<class "Scope5782_six_channel.lvclass">)  [unwired: 8 in, 1 out]
            n462 = call "WriteSetting 16bit.vi"("value"="Host scale", "FPGA Setting"=fpga_settings."Host scale", "FpgaRefBase in"=w739) -> ()  [unwired: 7 in, 2 out]
          }
          event "dw LP filter cut off frequency": Value Change {
            n463 = event-data() -> ()  [unwired: 1 in, 6 out]
            n464 = call "Read FpgaRef5761.vi"("Scope5785_six_channel"=w743) -> ("FpgaRef5761.lvclass"=w745:refnum<class "FpgaRef5761.lvclass">, "Scope5785_six_channel Out"=w742:refnum<class "Scope5782_six_channel.lvclass">)  [unwired: 8 in, 1 out]
            n465 = call "Write dw LP IIR coeffs.vi"("Fs [MHz}"=10.0, "cutoff fequency [MHz]"="dw LP filter cut off frequency", "FpgaRef5761"=w745) -> ()  [unwired: 8 in, 1 out]
          }
          event "Vi Vq LP  filter cutoff fequency": Value Change {
            n466 = event-data() -> ()  [unwired: 1 in, 6 out]
            n467 = call "Read FpgaRef5761.vi"("Scope5785_six_channel"=w750) -> ("FpgaRef5761.lvclass"=w751:refnum<class "FpgaRef5761.lvclass">, "Scope5785_six_channel Out"=w749:refnum<class "Scope5782_six_channel.lvclass">)  [unwired: 8 in, 1 out]
            n468 = call "Write Vi Vq IIR LP coeffs.vi"("Fs [MHz}"=10.0, "cutoff fequency [MHz]"="Vi Vq LP  filter cutoff fequency", "FpgaRef5761"=w751) -> ()  [unwired: 8 in, 1 out]
          }
          event "Vfi Vfq LP filter cut off frequency": Value Change {
            n469 = event-data() -> ()  [unwired: 1 in, 6 out]
            n470 = call "Read FpgaRef5761.vi"("Scope5785_six_channel"=w756) -> ("FpgaRef5761.lvclass"=w757:refnum<class "FpgaRef5761.lvclass">, "Scope5785_six_channel Out"=w755:refnum<class "Scope5782_six_channel.lvclass">)  [unwired: 8 in, 1 out]
            n471 = call "Write Vfi Vfq IIR LP coeffs.vi"("Fs [MHz}"=10.0, "cutoff fequency [MHz]"="Vfi Vfq LP filter cut off frequency", "FpgaRef5761"=w757) -> ()  [unwired: 8 in, 1 out]
          }
          event "w12 LP  filter cutoff fequency": Value Change {
            n472 = event-data() -> ()  [unwired: 1 in, 6 out]
            n473 = call "Read FpgaRef5761.vi"("Scope5785_six_channel"=w762) -> ("FpgaRef5761.lvclass"=w763:refnum<class "FpgaRef5761.lvclass">, "Scope5785_six_channel Out"=w761:refnum<class "Scope5782_six_channel.lvclass">)  [unwired: 8 in, 1 out]
            n474 = call "Write w12 LP IIR coeffs.vi"("Fs [MHz}"=10.0, "cutoff fequency [MHz]"="w12 LP  filter cutoff fequency", "FpgaRef5761"=w763) -> ()  [unwired: 8 in, 1 out]
          }
          event "ch1 delay", "ch3 delay": Value Change {
            n475 = event-data() -> ()  [unwired: 1 in, 6 out]
            n476 = local read "Mixer freq [MHz]"() -> (w778:dbl)
            n477 = Multiply(x="ch1 delay", y=0.001) -> (x*y=w779:dbl)
            n478 = Multiply(x="ch3 delay", y=0.001) -> (x*y=w780:dbl)
            n479 = call "Read FpgaRef5761.vi"("Scope5785_six_channel"=w769) -> ("FpgaRef5761.lvclass"=w775:refnum<class "FpgaRef5761.lvclass">, "Scope5785_six_channel Out"=w768:refnum<class "Scope5782_six_channel.lvclass">)  [unwired: 8 in, 1 out]
            n480 = Multiply(x=w778, y=6.283185307179586) -> (x*y=w776:dbl)
            n481 = Multiply(x=w779, y=w776) -> (x*y=w770:dbl)
            n482 = Multiply(x=w776, y=w780) -> (x*y=w773:dbl)
            n483 = call "WriteSetting float.vi"("value"=w770, "FPGA Setting"=fpga_settings."Fi_start", "FpgaRefBase in"=w775) -> ("FpgaRefBase out"=w774:refnum<class "FpgaRef5761.lvclass">)  [unwired: 7 in, 1 out]
            n484 = call "WriteSetting float.vi"("value"=w773, "FPGA Setting"=fpga_settings."Fi_delta", "FpgaRefBase in"=w774) -> ()  [unwired: 7 in, 2 out]
          }
          event "Update once upper", "Update once lower": Value Change {
            n485 = event-data() -> ()  [unwired: 1 in, 6 out]
            n486 = call "Write Update once lower.vi"("Update once lower"="Update once lower", "Scope5761"=w788) -> ("Scope5761"=w787:refnum<class "Scope5782_six_channel.lvclass">)  [unwired: 8 in, 1 out]
            n487 = call "Write Update once upper.vi"("Update once upper"="Update once upper", "Scope5761"=w787) -> ("Scope5761"=w786:refnum<class "Scope5782_six_channel.lvclass">)  [unwired: 8 in, 1 out]
          }
          event "Hold plot upper", "Hold plot lower": Value Change {
            w798 = T27."Enabled" ("Disabled")
            w797 = T27."Disabled and Grayed Out" ("Disabled")
            n488 = event-data() -> ()  [unwired: 1 in, 6 out]
            n489 = call "Write Hold plot upper.vi"("Hold plot upper"="Hold plot upper", "Scope5761"=w794) -> ("Scope5761"=w793:refnum<class "Scope5782_six_channel.lvclass">)  [unwired: 8 in, 1 out]
            n490 = call "Write Hold plot lower.vi"("Hold plot lower"="Hold plot lower", "Scope5761"=w793) -> ("Scope5761"=w792:refnum<class "Scope5782_six_channel.lvclass">)  [unwired: 8 in, 1 out]
            n491 = Select(t=w798, s="Hold plot upper", f=w797) -> (s? t:f=w791:T27)
            n492 = Select(t=w798, s="Hold plot lower", f=w797) -> (s? t:f=w790:T27)
            n493 = property on="Update once lower" class="Bool (strict)"("DisabledEnum"=w790) -> ()  [unwired: 2 in, 2 out]
            n494 = property on="Update once upper" class="Bool (strict)"("DisabledEnum"=w791) -> ()  [unwired: 2 in, 2 out]
          }
          event "Tau set", "Enable", "Measure Tau at Time", "Max output set": Value Change {
            n495 = event-data() -> ()  [unwired: 1 in, 6 out]
            n496 = Boolean To (0,1)(Boolean="Enable") -> (0, 1=w819:i16)
            n497 = Divide(x="Tau set", y=fxp<+/-,32,13> 6.399999618530273) -> (x/y=w818:fxp<+/-,32,13>)
            n498 = To Word Integer(number=w819) -> (16bit integer=w820:i16)
            n499 = xnode "Reinterpret Number"("x"=w818) -> ("y"=w823:fxp<+,32,32>)
            n500 = xnode "Reinterpret Number"("x"=w820) -> ("y"=w821:fxp<+/-,16,14>)
            n501 = To Fixed-Point(fixed-point type=fxp<+,16,14> 0.0, number="Max output set") -> (fixed-point=w805:fxp<+,16,14>)
            n502 = To Unsigned Long Integer(number=w823) -> (unsigned 32bit integer=w808:u32)
            n503 = xnode "Reinterpret Number"("x"=w821) -> ("y"=w809:fxp<+,16,16>)
            n504 = call "Write Setting 32bit.vi"("value"="Measure Tau at Time", "FPGA Setting"=fpga_settings."Quench t0", "ScopeBase in"=w815) -> ("ScopeBase out"=w814:refnum<class "Scope5782_six_channel.lvclass">)  [unwired: 7 in, 1 out]
            n505 = xnode "Reinterpret Number"("x"=w805) -> ("y"=w800:fxp<+,16,16>)
            n506 = call "Write Setting 32bit.vi"("value"=w808, "FPGA Setting"=fpga_settings."Quench tau set", "ScopeBase in"=w814) -> ("ScopeBase out"=w813:refnum<class "Scope5782_six_channel.lvclass">)  [unwired: 7 in, 1 out]
            n507 = call "Write Setting 16bit.vi"("value"=w809, "FPGA Setting"=fpga_settings."Quench enabled", "ScopeBase in"=w813) -> ("ScopeBase out"=w803:refnum<class "Scope5782_six_channel.lvclass">)  [unwired: 7 in, 1 out]
            n508 = call "Write Setting 16bit.vi"("value"=w800, "FPGA Setting"=fpga_settings."Quench max output", "ScopeBase in"=w803) -> ("ScopeBase out"=w801:refnum<class "Scope5782_six_channel.lvclass">)  [unwired: 7 in, 1 out]
          }
          event "Reset Quench Warning": Value Change {
            n509 = event-data() -> ()  [unwired: 1 in, 6 out]
            n510 = Boolean To (0,1)(Boolean="Reset Quench Warning") -> (0, 1=w832:i16)
            n511 = To Word Integer(number=w832) -> (16bit integer=w831:i16)
            n512 = xnode "Reinterpret Number"("x"=w831) -> ("y"=w830:fxp<+/-,16,14>)
            n513 = xnode "Reinterpret Number"("x"=w830) -> ("y"=w826:fxp<+,16,16>)
            n514 = call "Write Setting 16bit.vi"("value"=w826, "FPGA Setting"=fpga_settings."Quench reset", "ScopeBase in"=w828) -> ("ScopeBase out"=w827:refnum<class "Scope5782_six_channel.lvclass">)  [unwired: 7 in, 1 out]
          }
          event "Calculate w12": Value Change {
            n515 = event-data() -> ()  [unwired: 1 in, 6 out]
            n516 = call "Read FpgaRef5761.vi"("Scope5785_six_channel"=w837) -> ("FpgaRef5761.lvclass"=w836:refnum<class "FpgaRef5761.lvclass">, "Scope5785_six_channel Out"=w834:refnum<class "Scope5782_six_channel.lvclass">)  [unwired: 8 in, 1 out]
            n517 = call "SetW12Enabled.vi"("w12 enabled"="Calculate w12", "FpgaRef5761 In"=w836) -> ()  [unwired: 8 in, 2 out]
          }
          event "a", "b", "Fequency [kHz]": Value Change {
            n518 = event-data() -> ()  [unwired: 1 in, 6 out]
            n519 = call "SetAmPhase.vi"("b_am"="b", "a_am"="a", "fclk (MHz)"=100.0, "Am freq [kHz]"="Fequency [kHz]", "Scope5785_six_channel"=w844) -> ("Scope5785_six_channel out"=w843:refnum<class "Scope5782_six_channel.lvclass">)  [unwired: 5 in, 1 out]
          }
          event "w12 - b", "w12 - a", "w12 - dt": Value Change {
            n520 = event-data() -> ()  [unwired: 1 in, 6 out]
            n521 = To Fixed-Point(fixed-point type=fxp<+/-,32,12> 0.0 ("x"), number="w12 - a") -> (fixed-point=w864:fxp<+/-,32,12>)
            n522 = To Fixed-Point(fixed-point type=fxp<+/-,32,14> 0.0 ("x"), number="w12 - b") -> (fixed-point=w862:fxp<+/-,32,14>)
            n523 = To Fixed-Point(fixed-point type=fxp<+/-,32,26> 0.0 ("x"), number="w12 - dt") -> (fixed-point=w854:fxp<+/-,32,26>)
            n524 = call "Read FpgaRef5761.vi"("Scope5785_six_channel"=w847) -> ("FpgaRef5761.lvclass"=w868:refnum<class "FpgaRef5761.lvclass">, "Scope5785_six_channel Out"=w846:refnum<class "Scope5782_six_channel.lvclass">)  [unwired: 8 in, 1 out]
            n525 = xnode "Reinterpret Number"("x"=w864) -> ("y"=w865:fxp<+,32,32>)
            n526 = xnode "Reinterpret Number"("x"=w862) -> ("y"=w861:fxp<+,32,32>)
            n527 = xnode "Reinterpret Number"("x"=w854) -> ("y"=w855:fxp<+,32,32>)
            n528 = To Unsigned Long Integer(number=w865) -> (unsigned 32bit integer=w863:u32)
            n529 = To Unsigned Long Integer(number=w861) -> (unsigned 32bit integer=w857:u32)
            n530 = To Unsigned Long Integer(number=w855) -> (unsigned 32bit integer=w852:u32)
            n531 = call "WriteSetting 32bit.vi"("value"=w863, "FPGA Setting"=fpga_settings."w12_a", "FpgaRefBase in"=w868) -> ("FpgaRefBase out"=w859:refnum<class "FpgaRef5761.lvclass">)  [unwired: 7 in, 1 out]
            n532 = call "WriteSetting 32bit.vi"("value"=w857, "FPGA Setting"=fpga_settings."w12_b", "FpgaRefBase in"=w859) -> ("FpgaRefBase out"=w851:refnum<class "FpgaRef5761.lvclass">)  [unwired: 7 in, 1 out]
            n533 = call "WriteSetting 32bit.vi"("value"=w852, "FPGA Setting"=fpga_settings."w12_dt", "FpgaRefBase in"=w851) -> ()  [unwired: 7 in, 2 out]
          }
          event Value Change {
            n534 = event-data() -> ()  [unwired: 1 in, 6 out]
            n535 = call "Read FpgaRef5761.vi"("Scope5785_six_channel"=w877) -> ("FpgaRef5761.lvclass"=w874:refnum<class "FpgaRef5761.lvclass">, "Scope5785_six_channel Out"=w876:refnum<class "Scope5782_six_channel.lvclass">)  [unwired: 8 in, 1 out]
            n536 = To Unsigned Long Integer(number="w12 scale") -> (unsigned 32bit integer=w875:u32)
            n537 = To Unsigned Long Integer(number="dw scale") -> (unsigned 32bit integer=w871:u32)
            n538 = call "WriteSetting 32bit.vi"("value"=w875, "FPGA Setting"=fpga_settings."w12_scale", "FpgaRefBase in"=w874) -> ("FpgaRefBase out"=w872:refnum<class "FpgaRef5761.lvclass">)  [unwired: 7 in, 1 out]
            n539 = call "WriteSetting 32bit.vi"("value"=w871, "FPGA Setting"=fpga_settings."dw_scale", "FpgaRefBase in"=w872) -> ()  [unwired: 7 in, 2 out]
          }
        }
        n540 = case shown="False" w220 {
          tunnel: w219 -> [w230 _]
          frame False {
            n541 = Generate User Event(user event=w230, event data cluster=T25 {"Automatic"=TRUE, "Save"=TRUE} ("event data")) -> ()  [unwired: 2 in, 2 out]
          }
          frame True {
          }
        }
      }
      "stop 2" <- w208
    }
    frame Error {
    }
  }
  n542 = call "Run.vi"("SettingsFile in"=w14) -> ()  [unwired: 10 in, 1 out]
  n543 = Close Reference(reference=w44) -> ()  [unwired: 1 in, 1 out]
  n544 = Unregister For Events(event registration refnum=w134) -> ()  [unwired: 1 in, 1 out]
  n545 = call-dynamic "Close.vi"("ScopeBase in"=w103) -> ("error out"=w102:errorcluster)  [unwired: 10 in]
  n546 = flat-sequence {
    tunnel: w102 -> [_]
    frame #0 {
      n547 = global write "global_stop.vi" "Stop"(TRUE ("Stop")) -> ()
    }
  }
